vi "STED Control V13.vi"() -> ()   [LabVIEW 2014]
uses:
  Type Defs/Image Acquisition Parameters.ctl
  Laser Controls.ctl
  Detectors.ctl
  Type Defs/P541.ctl
  Type Defs/M227.ctl
  Type Defs/P612.ctl
  Type Defs/M686.ctl
  Type Defs/P841.ctl
  Type Defs/ASI.ctl
  Type Defs/N664_V2.ctl
  Type Defs/STED Graph Controls.ctl
  Type Defs/Display Controls.ctl
  Type Defs/Z comp.ctl
  FPGA-7842R-Reference.ctl
  Manual Controls V2.ctl
  Scan Parameters.ctl
  <vilib>/Utility/miscctls.llb/LVPositionTypeDef.ctl
  Controls/StageStates.ctl
  DM_Dual_V2/Controls/Standard Action.ctl
  Focus Lock/Controls/Counter Action.ctl
  Focus Lock/Controls/Standard Action for Focus Lock.ctl
  <vilib>/Utility/miscctls.llb/LVRectTypeDef.ctl
  <vilib>/event_ctls.llb/lveventtype.ctl
  <vilib>/Utility/file.llb/Read From Spreadsheet File (DBL).vi
  <vilib>/Utility/file.llb/Write To Spreadsheet File (DBL).vi
panel:
  in  "z Comp.":T1
  out "Graph Ref Out":refnum<vi>[](array[refnum])
  out "Frame Counter":i32
  in  "Follow Cursor":bool
  in  "Laser Controls 2":T2={"Laser On Time (Ticks)"=16, "Laser Delay (Ticks)"=3}
  out "Channel 6":sgl[][](graph)
  out "Channel 5":sgl[][](graph)
  out "Channel 4":sgl[][](graph)
  out "Channel 3":sgl[][](graph)
  out "Channel 2":sgl[][](graph)
  out "Channel 1":sgl[][](graph)
  in  "Display Controls":T3
  in  "Graph Tools":T4={"Zoom Out"=FALSE, "Zoom In"=FALSE, "Reset Zoom"=FALSE, "Pan Tool"=FALSE, "Show Cursor"=FALSE, "Load File"=FALSE, "Fit Tool"=FALSE, "Smooth Tool"=FALSE, "Merge Tool"=FALSE, "Auto Scale"=FALSE, "Apply Color"=FALSE, "Color Map"=enum."Fire"}
  in  "Shutters":T5
  in  "Upper Objective Z - N664":T6={"Up N664"=FALSE, "Down N664"=FALSE, "Step Size (um)"=0.001, "Position (mm)"=0.0, "Home"=FALSE, "Save"=FALSE} {"Step Size (um)" min=0.001}
  in  "Cavity Translation Z - ASI":T7={"Up ASI"=FALSE, "Down ASI"=FALSE, "Step Size (um)"=0.001, "Z (um)"=0.001, "F (um)"=0.001, "Velocity"=0.001} caption="ASI" {"Velocity" min=0.001; "F (um)" min=0.001; "Z (um)" min=-1500.0 max=1500.0; "Step Size (um)" min=0.001}
  in  "Phase Comp Mirror - P841":T8={"Position (µm)"=0.0, "Step Size (µm)"=0.05, "Up P841"=FALSE, "Down P841"=FALSE}
  in  "Sample Stage XY - M686":T9={"Home Button"=FALSE, "Up Button"=FALSE, "Left Button"=FALSE, "Down Button"=FALSE, "Right Button"=FALSE, "X"=0.0, "Y"=0.0, "Step Size (um)"=1.0} {"Y" format="%#_8g"; "X" format="%#_8g"}
  in  "Bottom Objective XY - P612":T10
  in  "Abort AllStage":bool
  in  "Stages":T11={"M227"=TRUE, "N664"=TRUE, "P612"=TRUE, "M686"=TRUE, "P841"=TRUE, "ASI"=FALSE}
  in  "Sample Z Coarse - M227":T12
  in  "Tab Control":T13(tab)
  in  "SLM":bool
  in  "DM":bool
  in  "Timing":bool
  in  "Focus Lock":bool
  in  "Stage Monitor":bool
  in  "Camera":bool
  in  "Sample Z - P541":T14={"Step Up"=FALSE, "Step Down"=FALSE, "Z Position"=0.0, "Step Size (um)"=1.0, "Home"=FALSE, "Save"=FALSE}
  in  "Detectors":T15={"PMT"=TRUE, "Far Red (685/40 nm)"=FALSE, "Orange (624/40 nm)"=FALSE, "Green (525/50 nm)"=FALSE, "Sum All"=FALSE}
  in  "Laser Controls":T16 {"STED Power (V)" scale=0.0..10.0}
  in  "Save File Path":path=path "C:/isoSTED_Data/Temp/Test_0000.dbl"
  in  "Capture":bool
  in  "Image Acquisition Parameters":T17={"Scan Type"=enum."Beam Scanning", "Scan Mode"=enum."XY", "Fast Axis Frequency (Hz)"=15780.0, "Image Format"=256, "Line Accumulations"=100, "Frames Per Capture"=1, "Frames Accumulations"=1, "Image Dimension (um)"=[15.0, 15.0], "Number of Z Steps"=1, "Z Steps Size (um)"=1.0, "Pixel Size (nm)"=[58.59375, 58.59375], "Customized Image Format"=[]} {"Z Steps Size (um)" min=0.0; "Number of Z Steps" min=1; "Frames Accumulations" min=1; "Frames Per Capture" min=1; "Line Accumulations" min=1; "Image Format" items=["64 x 64"=64, "128 x 128"=128, "256 x 256"=256, "512 x 512"=512, "1024 x 1024"=1024, "2048 x 2048"=2048, "Customized..."=0]}
  in  "Live":bool
  in  "Exit":bool
  # "Piston"
  # "Defocus"
  # "Length"
  # "Height"
  # "XY"
  # "Z"
  # "Length"
  # "Height"
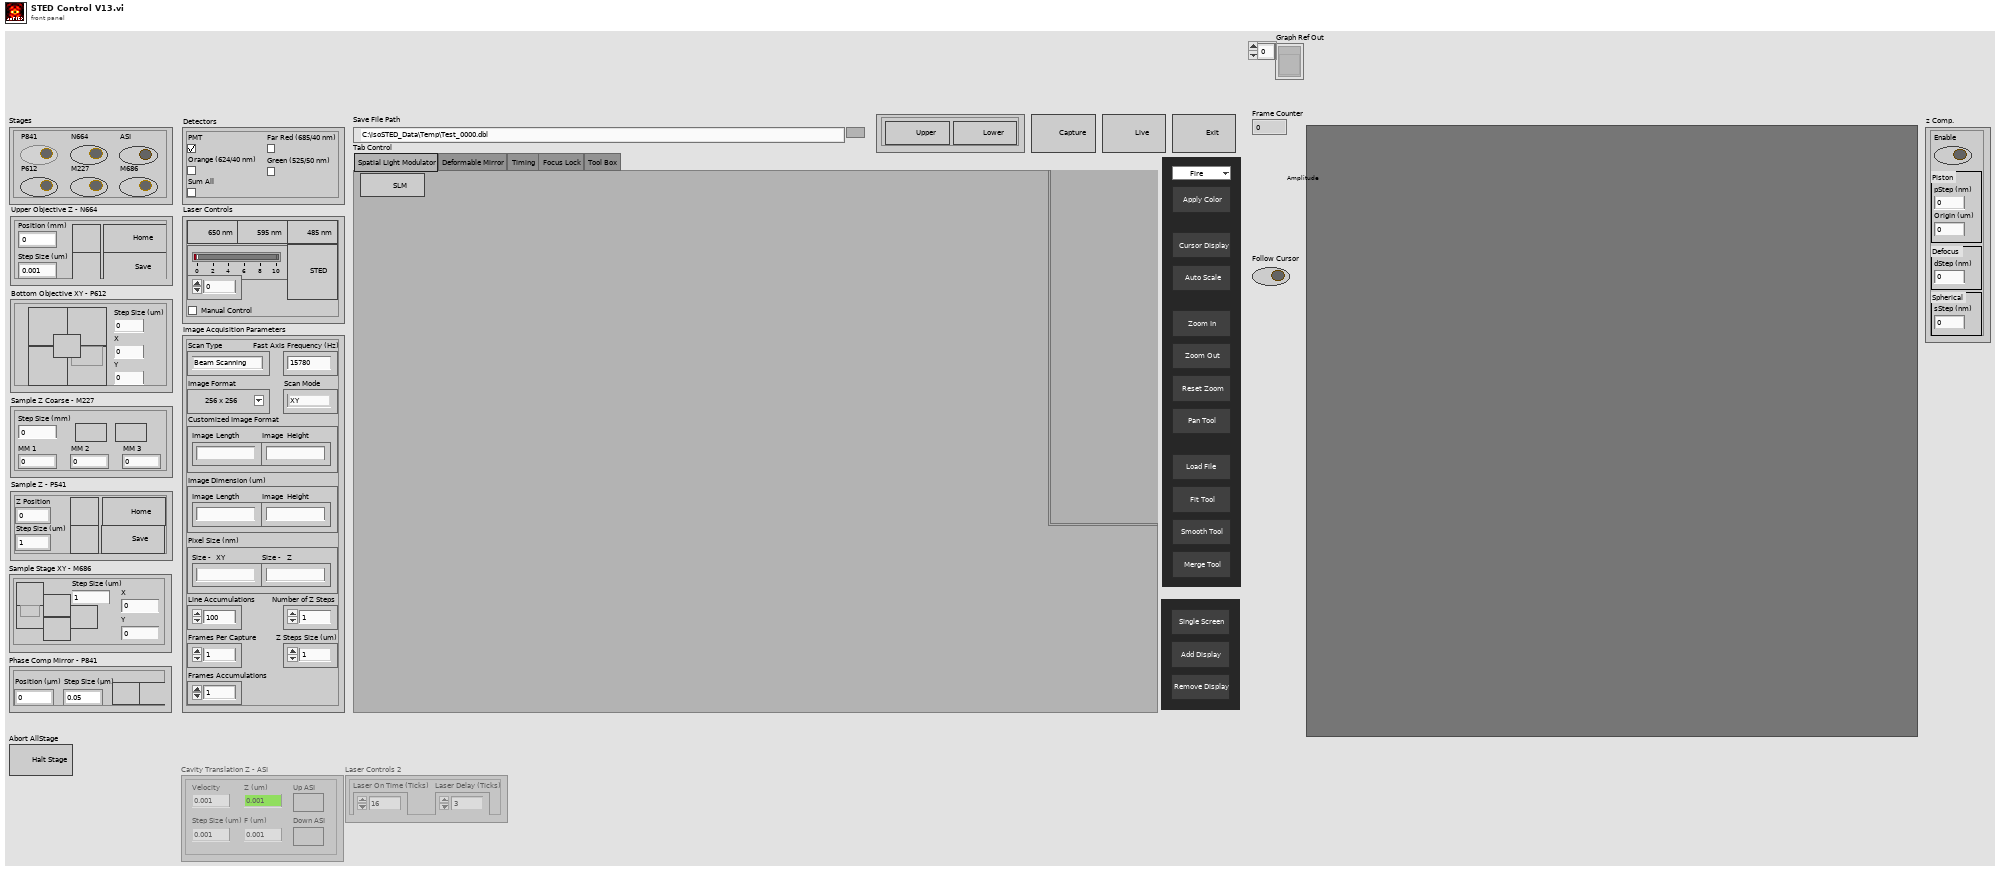
[diagram p1: front panel]
types:
  T1 = typedef "Z comp.ctl" = cluster{"Enable":bool, "pStep (nm)":dbl, "Origin (um)":dbl, "dStep (nm)":dbl, "sStep (nm)":dbl}
  T2 = cluster{"Laser On Time (Ticks)":i8, "Laser Delay (Ticks)":i8}
  T3 = typedef "Display Controls.ctl" = cluster{"Remove Display":bool, "Add Display":bool, "Single Screen":bool}
  T4 = typedef "STED Graph Controls.ctl" = cluster{"Zoom Out":bool, "Zoom In":bool, "Reset Zoom":bool, "Pan Tool":bool, "Show Cursor":bool, "Load File":bool, "Fit Tool":bool, "Smooth Tool":bool, "Merge Tool":bool, "Auto Scale":bool, "Apply Color":bool, "Color Map":enum16{"System", "Fire", "Gray", "Red", "Green", "Blue", "Cyan", "Magenta", "Yellow", "Red-White", "Green-White", "Blue-White", "Glow"}}
  T5 = cluster{"Upper Shutter":bool, "Lower Shutter":bool}
  T6 = typedef "N664_V2.ctl" = cluster{"Up N664":bool, "Down N664":bool, "Step Size (um)":dbl, "Position (mm)":dbl, "Home":bool, "Save":bool}
  T7 = typedef "ASI.ctl" = cluster{"Up ASI":bool, "Down ASI":bool, "Step Size (um)":dbl, "Z (um)":dbl, "F (um)":dbl, "Velocity":dbl}
  T8 = typedef "P841.ctl" = cluster{"Position (µm)":dbl, "Step Size (µm)":dbl, "Up P841":bool, "Down P841":bool}
  T9 = typedef "M686.ctl" = cluster{"Home Button":bool, "Up Button":bool, "Left Button":bool, "Down Button":bool, "Right Button":bool, "X":dbl, "Y":dbl, "Step Size (um)":dbl}
  T10 = typedef "P612.ctl" = cluster{"Home Button":bool, "Up Button":bool, "Left Button":bool, "Down Button":bool, "Right Button":bool, "Step Size (um)":dbl, "X":dbl, "Y":dbl}
  T11 = cluster{"M227":bool, "N664":bool, "P612":bool, "M686":bool, "P841":bool, "ASI":bool}
  T12 = typedef "M227.ctl" = cluster{"Up M227":bool, "Down M227":bool, "Step Size (mm)":dbl, "MM 1":dbl, "MM 2":dbl, "MM 3":dbl}
  T13 = enum32{"Spatial Light Modulator", "Deformable Mirror", "Timing", "Focus Lock", "Tool Box"}
  T14 = typedef "P541.ctl" = cluster{"Step Up":bool, "Step Down":bool, "Z Position":dbl, "Step Size (um)":dbl, "Home":bool, "Save":bool}
  T15 = typedef "Detectors.ctl" = cluster{"PMT":bool, "Far Red (685/40 nm)":bool, "Orange (624/40 nm)":bool, "Green (525/50 nm)":bool, "Sum All":bool}
  T16 = typedef "Laser Controls.ctl" = cluster{"STED Power (V)":dbl, "STED":bool, "650 nm":bool, "590 nm":bool, "485 nm":bool, "Manual Control":bool}
  T17 = typedef "Image Acquisition Parameters.ctl" = cluster{"Scan Type":enum16{"Sample Scanning", "Beam Scanning"}, "Scan Mode":enum16{"XY", "XZ", "YZ", "XYZ"}, "Fast Axis Frequency (Hz)":dbl, "Image Format":u16, "Line Accumulations":u16, "Frames Per Capture":u16, "Frames Accumulations":u16, "Image Dimension (um)":dbl[], "Number of Z Steps":u8, "Z Steps Size (um)":dbl, "Pixel Size (nm)":dbl[], "Customized Image Format":dbl[]}
  T18 = typedef "Scan Parameters.ctl" = cluster{"Fast_Ax_Amp_V":dbl, "Fast_Ax_Off_V":dbl, "Slow_Ax_Amp_V":dbl, "Slow_Ax_Off_V ":dbl, "Slow_Ax_Max_V_VperS":dbl, "Slow_Ax1_Del25ns":i32, "Slow_Ax2_Del25ns":i32, "Stage_X_Off_V":dbl, "Stage_Y_Off_V":dbl, "Stage_Z_Off_V":dbl, "Galvo1_Off_V":dbl, "Galvo2_Off_V":dbl, "Last_Scan_Mode":enum16{"XY", "XZ", "YZ", "XYZ"}, "Current_Scan_Mode":enum16{"XY", "XZ", "YZ", "XYZ"}, "Fly_Back_Lines":u16, "Linear_Ramp_End":u32, "Z_Step_I16":i16, "Z_Start_I16":i16, "Laser_States _U32":u32, "590_Voltage_I16":i16, "775_AOM_Volt_I16":i16, "Blanking OFF":bool, "Unused_Axis_I16":i16}
  T19 = typedef "Manual Controls V2.ctl" = cluster{"Galvo 1 Position (I16)":i16, "Galvo 2 Position (I16)":i16, "X Axis Voltage (I16)":i16, "Y Axis Voltage (I16)":i16, "Z Axis Voltage (I16)":i16, "Res Mirror Amp (I16)":i16, "Res Mirror Mute":bool, "Upper Shutter":bool, "Lower Shutter":bool}
  T20 = typedef "FPGA-7842R-Reference.ctl" = enum16{"Stage Control", "Laser Control", "Unused Axis I16", "Exit", "Set Res Mirror", "Set Galvo", "Current Frame for Capture", "Default", "Close FPGA", "Stop Waveforms", "Start Waveforms", "Shutter Control", "Initialize"}
  T21 = typedef "Counter Action.ctl" = enum16{"Zero", "Plus One", "Read"}
  T22 = typedef "StageStates.ctl" = enum16{"POSITION", "MVR", "MOVE", "HALT", "ONTARGET", "ERROR", "EXIT", "HOME", "ZEROPOS", "NANOPOS", "QUIT", "ANALOG"}
  T23 = enum8{"Enabled", "Disabled", "Disabled and Grayed Out"}
  T24 = typedef "Standard Action.ctl" = enum16{"Read", "Write"}
  T25 = typedef "Standard Action for Focus Lock.ctl" = enum16{"Read", "Write"}
  T26 = typedef "LVRectTypeDef.ctl" = cluster{"Left":i16, "Top":i16, "Right":i16, "Bottom":i16}
  T27 = enum32{"Invalid", "Standard", "Closed", "Hidden", "Minimized", "Maximized"}
  T28 = typedef "lveventtype.ctl" = enum32{"Null", "Timeout", "Annotation Menu Selection", "Annotation Menu Selection?", "App Instance Close", "App Instance Close?", "Autoscale Range Change", "Bookmark Info Change", "Cell Edit", "Cell Edit?", "Cursor Grab", "Cursor Grab?", "Cursor Menu Selection", "Cursor Menu Selection?", "Cursor Move", "Cursor Release", "Data Change", "Direction Change", "Display State Change", "Drag Ended", "Drag Enter", "Drag Leave", "Drag Over", "Drag Source Update", "Drag Starting", "Drag Starting?", "Drop", "Exec State Change", "Key Down", "Key Down?", "Key Repeat", "Key Repeat?", "Key Up", "Listbox Double Click", "Menu Activation?", "Menu Selection (App)", "Menu Selection? (App)", "Menu Selection (User)", "Mouse Down", "Mouse Down?", "Mouse Enter", "Mouse Leave", "Mouse Move", "Mouse Up", "Mouse Wheel", "NI Security User Change (App)", "Pane Size", "Panel Close", "Panel Close?", "Panel Resize", "Plot Attribute Change", "Scale Range Change", "Shortcut Menu Activation?", "Shortcut Menu Selection (App)", "Shortcut Menu Selection? (App)", "Shortcut Menu Selection (User)", "Tree Double Click", "Tree Drag", "Tree Drag?", "Tree Drop", "Tree Drop?", "Tree Item Close", "Tree Item Close?", "Tree Item Open", "Tree Item Open?", "User Event", "Value Change"}
  T29 = typedef "LVPositionTypeDef.ctl" = cluster{"Left":i32, "Top":i32}
  T30 = cluster{"Upper Shutter":bool, "Upper Shutter":bool}
  T31 = cluster{bool, bool, dbl, "Numeric":dbl, "Numeric":dbl, "Numeric":dbl}
  T32 = cluster{"Down_N664":bool, "Down_N664":bool, "Step Size (um)":dbl, "Numeric":dbl, bool, bool}
  T33 = cluster{bool, bool, bool, bool, bool, dbl, "Numeric":dbl, "Numeric":dbl}
  T34 = cluster{bool, bool, bool, bool, bool, "Numeric":dbl, "Numeric":dbl, dbl}
  T35 = cluster{"Enable":bool, "pStep (nm)":bool, "Origin (um)":bool, "dStep (nm)":bool, "sStep (nm)":bool}
  T36 = typedef "MirrorModes_DUAL.ctl" = cluster{"Mode":string, "Amplitude":dbl}[][]
  T37 = cluster{"Scan Type":bool, "Scan Mode":bool, "Fast Axis Frequency (Hz)":bool, "Image Format":bool, "Line Accumulations":bool, "Frames Per Capture":bool, "Frames Accumulations":bool, "Image Dimension (um)":bool[], "Number of Z Steps":bool, "Z Steps Size (um)":bool, "Pixel Size (nm)":bool[], "Customized Image Format":bool[]}
  T38 = typedef "Focus Lock.ctl" = cluster{"EXIT":bool, "Lock Current":bool, "Manual":bool, "Drift":bool, "Move":bool, "Control Option":bool}
  T39 = typedef "LVAllMonitorsDisplayTypeDef.ctl" = cluster{"Bounds":cluster{"Left":i16, "Top":i16, "Right":i16, "Bottom":i16}, "Depth":i16}[]
  T40 = cluster{"Bounds":cluster{"Left":i16, "Top":i16, "Right":i16, "Bottom":i16}, "Depth":i16}
  T41 = enum16{"System", "Fire", "Gray", "Red", "Green", "Blue", "Cyan", "Magenta", "Yellow", "Red-White", "Green-White", "Blue-White", "Glow"}
  T42 = typedef "LVPointDoubleTypeDef.ctl" = cluster{"Cursor X":dbl, "Cursor Y":dbl}
  T43 = typedef "LVRangeTypeDef.ctl" = cluster{"Minimum":dbl, "Maximum":dbl, "Increment":dbl, "Minor Increment":dbl, "Start":dbl}
  T44 = typedef "IMAQ Image.ctl" = refnum<image>
  T45 = typedef "Waveform Data.ctl" = cluster{"Waveform Scan Parameters":cluster{"Scanning Mode":u8, "Fast Axis WF Length (Elements)":i32, "Fast Axis Sample Period (Ticks)":u32, "Slow Axis 1 WF Length (Elements)":i32, "Slow Axis 1 Sample Period (Ticks)":u32, "Slow Axis 1 Delay (25 ns) Steps":i32, "Slow Axis 2 WFLength (Elements)":i32, "Slow Axis 2 Sample Period (Ticks)":u32, "Slow Axis 2 Delay (25 ns) Steps":i32}, "Fast Axis Waveform":dbl[], "Slow Axis 1 Waveform":dbl[], "Slow Axis 2 Waveform":dbl[]}
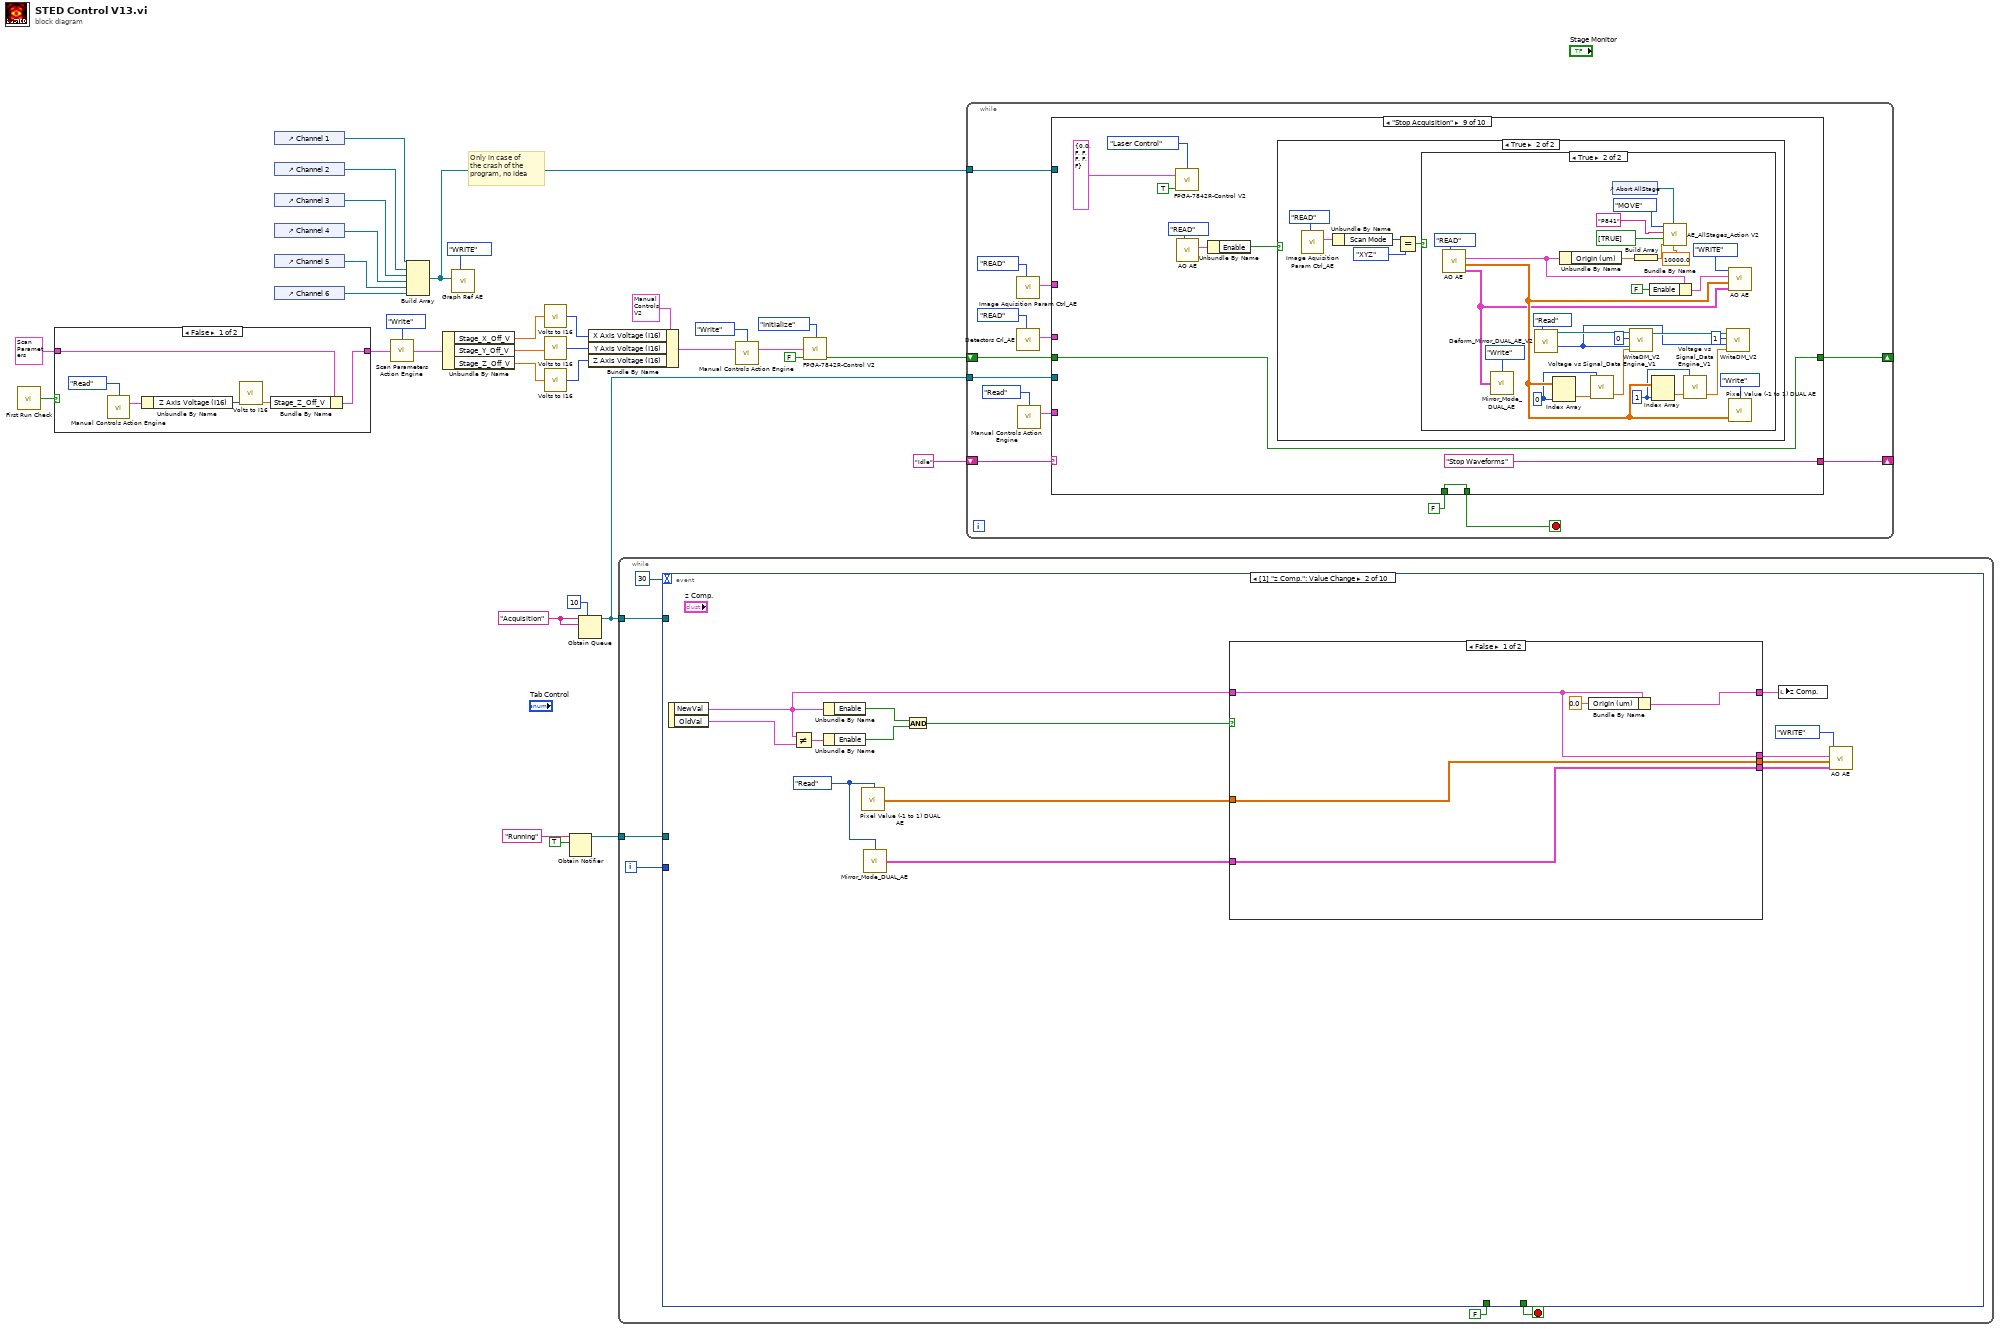
[diagram p0: block diagram]
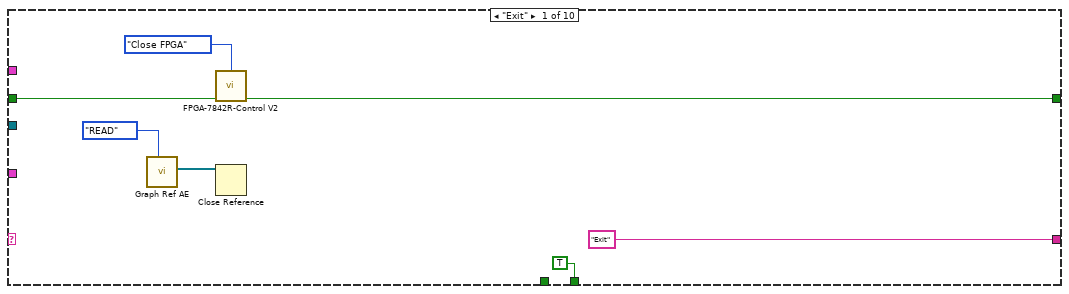
[diagram p3: hidden frame]
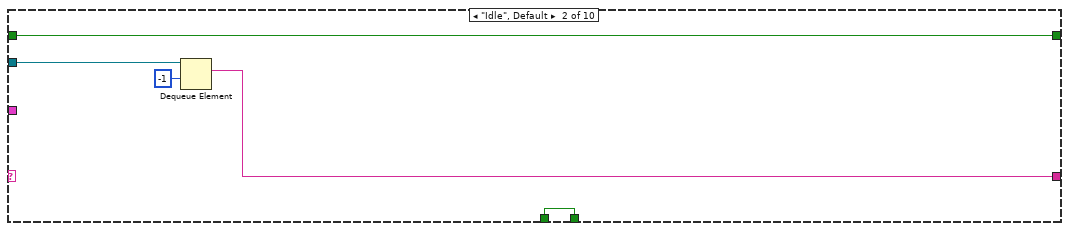
[diagram p4: hidden frame]
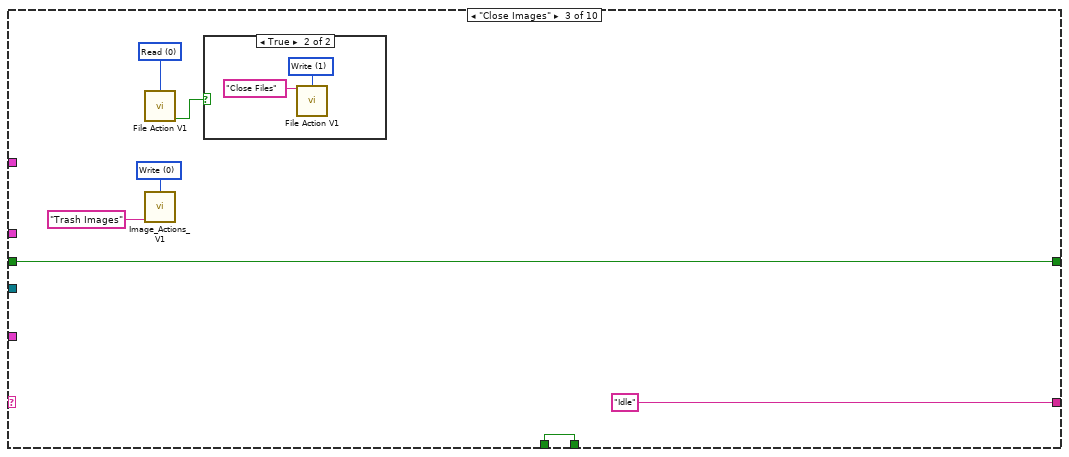
[diagram p5: hidden frame]
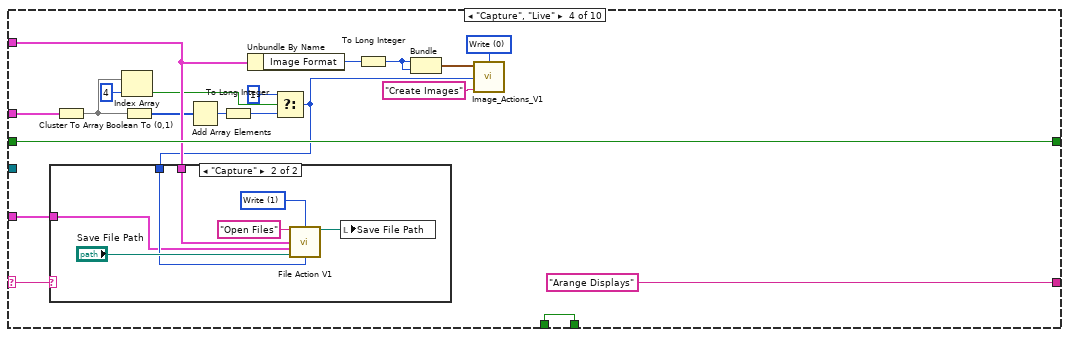
[diagram p7: hidden frame]
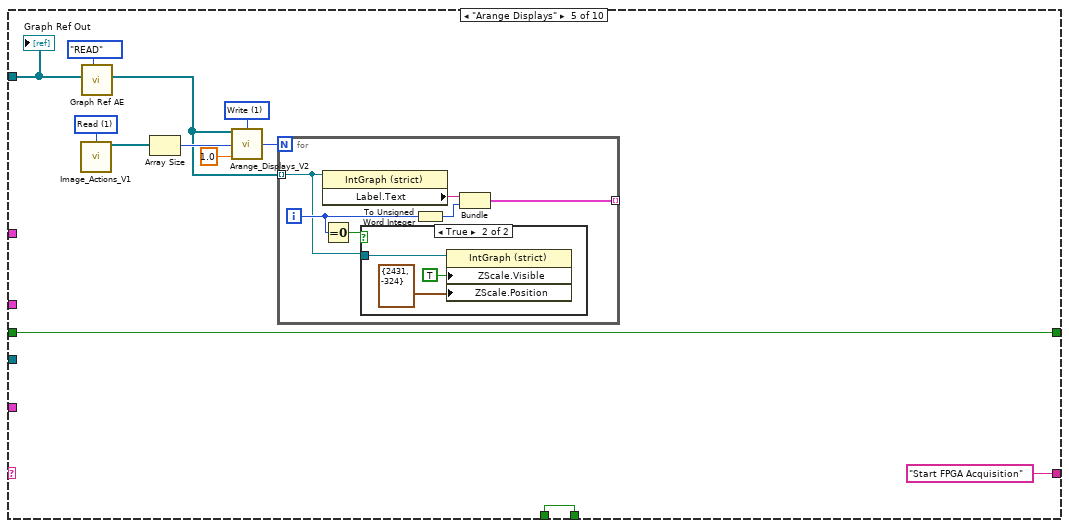
[diagram p9: hidden frame]
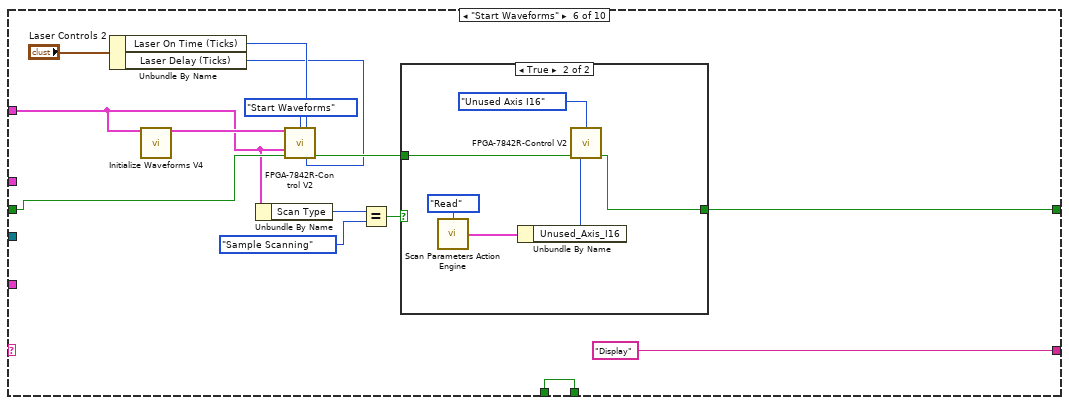
[diagram p11: hidden frame]
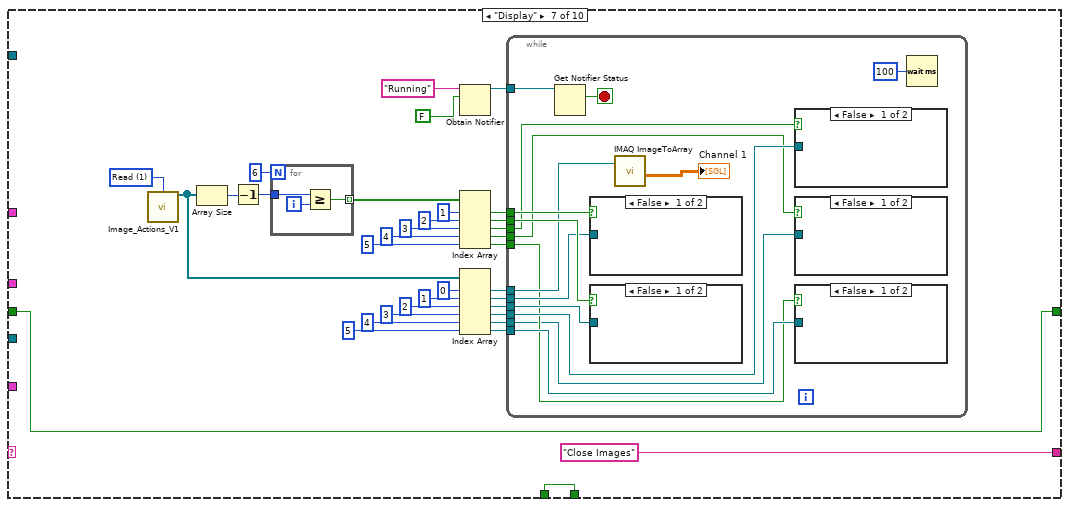
[diagram p13: hidden frame]
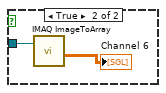
[diagram p14: hidden frame]
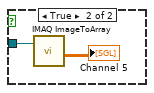
[diagram p15: hidden frame]
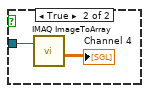
[diagram p16: hidden frame]
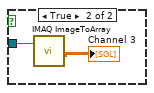
[diagram p17: hidden frame]
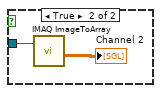
[diagram p18: hidden frame]
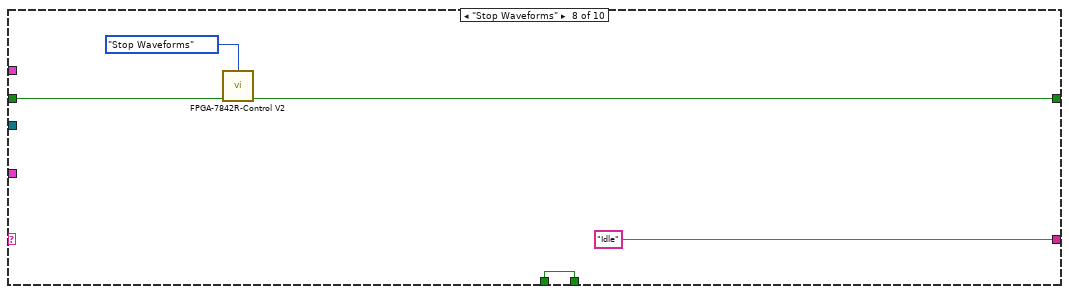
[diagram p19: hidden frame]
diagram:
  w16 = "Acquisition" ("name (unnamed)")
  # "Only in case of \nthe crash of the\nprogram, no idea"
  n1 = call "First Run Check.vi"() -> ("First Run?"=w10:bool)  [unwired: 15 in]
  n2 = case shown="False" w10 {
    tunnel: T18 {"Fast_Ax_Amp_V"=0.0, "Fast_Ax_Off_V"=0.0, "Slow_Ax_Amp_V"=0.0, "Slow_Ax_Off_V "=0.0, "Slow_Ax_Max_V_VperS"=0.0, "Slow_Ax1_Del25ns"=0, "Slow_Ax2_Del25ns"=0, "Stage_X_Off_V"=5.0, "Stage_Y_Off_V"=5.0, "Stage_Z_Off_V"=5.0, "Galvo1_Off_V"=0.0, "Galvo2_Off_V"=0.0, "Last_Scan_Mode"=enum."XY", "Current_Scan_Mode"=enum."XY", "Fly_Back_Lines"=0, "Linear_Ramp_End"=0, "Z_Step_I16"=0, "Z_Start_I16"=0, "Laser_States _U32"=0, "590_Voltage_I16"=0, "775_AOM_Volt_I16"=0, "Blanking OFF"=FALSE, "Unused_Axis_I16"=16384} ("Scan Parameters IN") -> [w39 w40]
    tunnel: [w34 w40] -> w8
    frame False {
      n3 = call "Manual Controls Action Engine.vi"("Action"=enum16{"Read", "Write"}."Read") -> ("Manual Controls Out"=w37:T19)  [unwired: 14 in]
      n4 = Unbundle By Name(w37) -> ("Z Axis Voltage (I16)"=w38:i16)
      n5 = call "Volts to I16.vi"("Volatge (I16)"=w38) -> ("Voltage (V)"=w35:dbl)  [unwired: 13 in, 1 out]
      n6 = Bundle By Name(cluster=w39, "Stage_Z_Off_V"=w35) -> (w34:T18)
    }
    frame True {
    }
  }
  n7 = control-ref of="Channel 1"() -> (w5:refnum<vi>)
  n8 = control-ref of="Channel 2"() -> (w6:refnum<vi>)
  n9 = control-ref of="Channel 3"() -> (w7:refnum<vi>)
  n10 = control-ref of="Channel 4"() -> (w2:refnum<vi>)
  n11 = control-ref of="Channel 5"() -> (w4:refnum<vi>)
  n12 = control-ref of="Channel 6"() -> (w3:refnum<vi>)
  n13 = call "Scan Parameters Action Engine.vi"("Action"=enum16{"Read", "Write"}."Write", "Scan Parameters IN"=w8) -> ("Scan Parameters OUT"=w26:T18)  [unwired: 13 in]
  n14 = Build Array(w5, w6, w7, w2, w4, w3) -> (w1:refnum<vi>[])
  n15 = Unbundle By Name(w26) -> ("Stage_X_Off_V"=w22:dbl, "Stage_Y_Off_V"=w21:dbl, "Stage_Z_Off_V"=w20:dbl)
  n16 = call "Graph Ref AE.vi"("Action"=enum16{"READ", "WRITE"}."WRITE", "Graph Ref In"=w1) -> ()  [unwired: 9 in, 1 out]
  n17 = call "Volts to I16.vi"("Voltage (V)"=w22) -> ("I16"=w23:i16)  [unwired: 13 in, 1 out]
  n18 = call "Volts to I16.vi"("Voltage (V)"=w21) -> ("I16"=w24:i16)  [unwired: 13 in, 1 out]
  n19 = call "Volts to I16.vi"("Voltage (V)"=w20) -> ("I16"=w25:i16)  [unwired: 13 in, 1 out]
  n20 = Obtain Notifier(name (unnamed)="Running", notification data type=TRUE) -> (notifier out=w12:refnum<notifier>)  [unwired: 2 in, 2 out]
  n21 = Obtain Queue(max queue size (-1, unlimited)=10, name (unnamed)=w16, element data type=w16) -> (queue out=w18:refnum<queue>)  [unwired: 2 in, 2 out]
  n22 = Bundle By Name(cluster=T19 {"Galvo 1 Position (I16)"=-280, "Galvo 2 Position (I16)"=0, "X Axis Voltage (I16)"=16384, "Y Axis Voltage (I16)"=16384, "Z Axis Voltage (I16)"=16384, "Res Mirror Amp (I16)"=0, "Res Mirror Mute"=FALSE, "Upper Shutter"=FALSE, "Lower Shutter"=FALSE} ("Manual Controls"), "X Axis Voltage (I16)"=w23, "Y Axis Voltage (I16)"=w24, "Z Axis Voltage (I16)"=w25) -> (w27:T19)
  n23 = while {
    tunnel: w18 -> [w44]
    tunnel: w12 -> [w41]
    i -> [w42]
    stop <- w46 stop-if-true
    n24 = event shown="[1] \"z Comp.\": Value Change" {
      selector: _ -> [_ _ _ _ _ _ _ _ _ _]
      dyn-events: _ -> [_ _ _ _ _ _ _ _ _ _]
      timeout: 30 -> [_ _ _ _ _ _ _ _ _ _]
      tunnel: [w54 _ w258 w302 w467 _ w814 w909 w1113 w1166] -> w46
      tunnel: FALSE -> [w54 _ w258 w302 w467 _ w814 w909 w1113 _]
      tunnel: w44 -> [w51 _ w257 _ _ _ _ _ _ w1165]
      tunnel: w42 -> [w49 _ _ _ _ _ _ _ _ _]
      tunnel: w41 -> [w47 _ w255 _ _ _ _ _ _ w1159]
      event Timeout {
        n25 = event-data() -> ()  [unwired: 1 in, 3 out]
        n26 = Equal To 0?(x=w49) -> (x = 0?=w48:bool)
        n27 = Get Notifier Status(notifier=w47) -> (current notification=w53:bool)  [unwired: 1 in, 4 out]
        n28 = case shown="False" w48 {
          frame False {
            w64 = enum16{"WRITE", "READ", "HOME", "SAVE HOME"}."READ" ("Enum")
            n29 = call "AO AE.vi"("Action"=enum16{"READ", "WRITE"}."READ") -> ("Z Comp. Output"=w57:T1)  [unwired: 8 in, 2 out]
            n30 = Unbundle By Name(w57) -> ("Enable"=w62:bool, "Origin (um)"=w58:dbl, "pStep (nm)"=w59:dbl, "dStep (nm)"=w56:dbl, "sStep (nm)"=w55:dbl)
            n31 = call "Image Aquisition Param Ctrl_AE.vi"("Action"=enum16{"READ", "WRITE"}."READ") -> ("Image Acquisition Parameters Out"=w98:T17)  [unwired: 10 in]
            n32 = call "Detectors Crl_AE.vi"("Action"=enum16{"READ", "WRITE"}."READ") -> ("Detectors Parameters Out"=w99:T15)  [unwired: 10 in]
            n33 = call "LASERs_ Crl_AE.vi"("Action"=enum16{"READ", "WRITE"}."READ") -> ("Detectors Parameters Out"=w100:T16)  [unwired: 10 in]
            n34 = local write "z Comp."(w57) -> ()
            n35 = local write "Image Acquisition Parameters"(w98) -> ()
            n36 = local write "Detectors"(w99) -> ()
            n37 = local write "Laser Controls"(w100) -> ()
            n38 = call "Frame Counter.vi"("Action"=Counter_Action."Read") -> ("Num"=w63:i32)
            "Frame Counter" <- w63
            n39 = case shown="True" w62 {
              tunnel: w63 -> [_ w104]
              tunnel: w59 -> [_ w105]
              tunnel: w58 -> [_ w103]
              tunnel: w57 -> [_ _]
              tunnel: w56 -> [_ w102]
              tunnel: w55 -> [_ w101]
              frame False {
              }
              frame True {
                n40 = local read "Capture"() -> (w112:bool)
                n41 = local read "Live"() -> (w113:bool)
                n42 = call "Image Aquisition Param Ctrl_AE.vi"("Action"=enum16{"READ", "WRITE"}."READ") -> ("Image Acquisition Parameters Out"=w114:T17)  [unwired: 10 in]
                n43 = Or(x=w112, y=w113) -> (x .or. y?=w109:bool)
                n44 = Unbundle By Name(w114) -> ("Scan Mode"=w111:enum16{"XY", "XZ", "YZ", "XYZ"}, "Number of Z Steps"=w106:u8)
                n45 = Equal?(x=enum16{"XY", "XZ", "YZ", "XYZ"}."XYZ", y=w111) -> (x = y?=w108:bool)
                n46 = And(x=w109, y=w108) -> (x .and. y?=w107:bool)
                n47 = case shown="True" w107 {
                  tunnel: w104 -> [_ w125]
                  tunnel: w106 -> [_ w124]
                  tunnel: w105 -> [_ w123]
                  tunnel: w103 -> [_ w122]
                  tunnel: w102 -> [_ w117]
                  tunnel: w101 -> [_ w116]
                  frame False {
                  }
                  frame True {
                    n48 = Quotient & Remainder(x=w125, y=w124) -> (x-y*floor(x/y)=w118:i32)  [unwired: 1 out]
                    n49 = control-ref of="Abort AllStage"() -> (w120:refnum<vi>)
                    n50 = call "Defocus and Spherical Comp V2.vi"("Spherical Step"=w116, "Defocus Step"=w117, "Step #"=w118) -> ()  [unwired: 1 in]
                    n51 = call "Piston Comp.vi"("Abort"=w120, "Step Size"=w123, "Step #"=w118, "Original Position"=w122, "Action"=enum16{"MOVE", "BACK TO ORIGINE"}."MOVE") -> ("position"=w119:dbl)  [unwired: 5 in]
                    n52 = property on="Position (µm)" class="DigNum (strict)"("Value"=w119) -> ()  [unwired: 2 in, 2 out]
                  }
                }
              }
            }
            n53 = call "Stage_position_ae.vi"("StageID"="M686", "Enum"=w64) -> ("Position Out"=w74:dbl[])  [unwired: 8 in, 1 out]
            n54 = call "Stage_position_ae.vi"("StageID"="M227", "Enum"=w64) -> ("Position Out"=w81:dbl[])  [unwired: 8 in, 1 out]
            n55 = call "Stage_position_ae.vi"("StageID"="N664", "Enum"=w64) -> ("Position Out"=w67:dbl[])  [unwired: 8 in, 1 out]
            n56 = call "Stage_position_ae.vi"("StageID"="P841", "Enum"=w64) -> ("Position Out"=w88:dbl[])  [unwired: 8 in, 1 out]
            n57 = call "Stage_position_ae.vi"("StageID"="P612", "Enum"=w64) -> ("Position Out"=w65:dbl[])  [unwired: 8 in, 1 out]
            n58 = Index Array(array=w67, index=0) -> (element=w84:dbl)
            n59 = Index Array(array=w88, index=0) -> (element=w61:dbl)
            n60 = Index Array(array=w65, index #1=0 ("index"), index #2=1 ("index"), index #3=2 ("index")) -> (element #1=w94:dbl, element #2=w91:dbl, element #3=w89:dbl)
            n61 = Index Array(array=w74, index #1=0 ("index"), index #2=1 ("index")) -> (element #1=w71:dbl, element #2=w70:dbl)
            n62 = Index Array(array=w81, index #1=0 ("index"), index #2=1 ("index"), index #3=2 ("index")) -> (element #1=w78:dbl, element #2=w77:dbl, element #3=w76:dbl)
            n63 = property on="Position (µm)" class="DigNum (strict)"("Value"=w61) -> ()  [unwired: 2 in, 2 out]
            n64 = property on="Position (mm)" class="DigNum (strict)"("Value"=w84) -> ()  [unwired: 2 in, 2 out]
            n65 = property on="X" class="DigNum (strict)"("Value"=w94) -> ()  [unwired: 2 in, 2 out]
            n66 = property on="Y" class="DigNum (strict)"("Value"=w91) -> ()  [unwired: 2 in, 2 out]
            n67 = property on="X" class="DigNum (strict)"("Value"=w71) -> ()  [unwired: 2 in, 2 out]
            n68 = property on="MM 1" class="DigNum (strict)"("Value"=w78) -> ()  [unwired: 2 in, 2 out]
            n69 = property on="MM 2" class="DigNum (strict)"("Value"=w77) -> ()  [unwired: 2 in, 2 out]
            n70 = property on="Z Position" class="DigNum (strict)"("Value"=w89) -> ()  [unwired: 2 in, 2 out]
            n71 = property on="Y" class="DigNum (strict)"("Value"=w70) -> ()  [unwired: 2 in, 2 out]
            n72 = property on="MM 3" class="DigNum (strict)"("Value"=w76) -> ()  [unwired: 2 in, 2 out]
          }
          frame True {
            w127 = FALSE ("SLM")
            w129 = enum16{"WRITE", "READ", "HOME", "SAVE HOME"}."SAVE HOME" ("Enum")
            w141 = FALSE ("Upper Shutter")
            n73 = local read "Image Acquisition Parameters"() -> (w148:T17)
            n74 = local read "Laser Controls"() -> (w146:T16)
            n75 = local read "Detectors"() -> (w145:T15)
            n76 = Bundle("Upper Shutter"=w141, "Upper Shutter"=w141) -> (w142:T30)  [unwired: 1 in]
            n77 = property on="Shutters" class="Clust (strict)"("Value"=w142) -> ()  [unwired: 2 in, 2 out]
            n78 = call "Image Aquisition Param Ctrl_AE.vi"("Action"=enum16{"READ", "WRITE"}."WRITE", "Image Acquisition Parameters In"=w148) -> ()  [unwired: 9 in, 1 out]
            n79 = call "Detectors Crl_AE.vi"("Action"=enum16{"READ", "WRITE"}."WRITE", "Detectors Parameters In"=w145) -> ()  [unwired: 9 in, 1 out]
            n80 = call "LASERs_ Crl_AE.vi"("Action"=enum16{"READ", "WRITE"}."WRITE", "Detectors Parameters In"=w146) -> ()  [unwired: 9 in, 1 out]
            n81 = property on="Stages" class="Clust (strict)"() -> ("Controls[]"=w143:refnum<vi>[])  [unwired: 2 in, 2 out]
            n82 = for {
              tunnel: w143 -> [w153] mode=indexing
              n83 = property class="Ctl"(reference=w153) -> ("Label.Text"=w151:string, "Value"=w155:variant)  [unwired: 1 in, 2 out]
              n84 = Variant To Data(type=TRUE, Variant=w155) -> (data=w152:bool)  [unwired: 1 in, 1 out]
              n85 = call "All_Stages_Aloha.vi"("Aloha"=w152, "Stage ID"=w151) -> ("Position Out"=w150:dbl[])  [unwired: 9 in]
              n86 = case shown="\"M686\"" w151 {
                tunnel: w150 -> [_ w162 w170 w177 w186 w197 w207]
                frame "0", Default {
                }
                frame "M227" {
                  w166 = FALSE
                  n87 = Index Array(array=w162, index #1=0 ("index"), index #2=1 ("index"), index #3=2 ("index")) -> (element #1=w158:dbl, element #2=w157:dbl, element #3=w156:dbl)
                  n88 = Bundle(w166, w166, 0.0, "Numeric"=w158, "Numeric"=w157, "Numeric"=w156) -> (w164:T31)  [unwired: 1 in]
                  n89 = To Variant(anything=w164) -> (Variant=w163:variant)
                  n90 = property on="Sample Z Coarse - M227" class="Clust"("Value"=w163) -> ()  [unwired: 2 in, 2 out]
                }
                frame "N664" {
                  w167 = FALSE
                  w173 = FALSE ("Down_N664")
                  n91 = Index Array(array=w170, index=0) -> (element=w171:dbl)
                  n92 = Bundle("Down_N664"=w173, "Down_N664"=w173, "Step Size (um)"=1.0, "Numeric"=w171, w167, w167) -> (w169:T32)  [unwired: 1 in]
                  n93 = To Variant(anything=w169) -> (Variant=w168:variant)
                  n94 = property on="Upper Objective Z - N664" class="Clust"("Value"=w168) -> ()  [unwired: 2 in, 2 out]
                }
                frame "P612" {
                  w185 = FALSE
                  n95 = Index Array(array=w177, index #1=0, index #2=1, index #3=2 ("index")) -> (element #1=w182:dbl, element #2=w180:dbl, element #3=w175:dbl)
                  n96 = Bundle(w185, w185, w185, w185, w185, 1.0, "Numeric"=w182, "Numeric"=w180) -> (w181:T33)  [unwired: 1 in]
                  n97 = To Variant(anything=w181) -> (Variant=w176:variant)
                  n98 = property on="Bottom Objective XY - P612" class="Clust"("Value"=w176) -> ()  [unwired: 2 in, 2 out]
                  n99 = property on="Z Position" class="DigNum (strict)"("Value"=w175) -> ()  [unwired: 2 in, 2 out]
                }
                frame "M686" {
                  w195 = FALSE
                  n100 = Index Array(array=w186, index #1=0, index #2=1) -> (element #1=w190:dbl, element #2=w189:dbl)
                  n101 = Bundle(w195, w195, w195, w195, w195, "Numeric"=w190, "Numeric"=w189, 1.0) -> (w193:T34)  [unwired: 1 in]
                  n102 = To Variant(anything=w193) -> (Variant=w191:variant)
                  n103 = property on="Sample Stage XY - M686" class="Clust"("Value"=w191) -> ()  [unwired: 2 in, 2 out]
                  n104 = call "M686_timer.vi"("Reset"=TRUE) -> ()  [unwired: 1 out]
                }
                frame "P841" {
                  n105 = Index Array(array=w197, index=0) -> (element=w196:dbl)
                  n106 = property on="Position (µm)" class="DigNum (strict)"("Value"=w196) -> ()  [unwired: 2 in, 2 out]
                }
                frame "ASI" {
                  w203 = FALSE
                  n107 = Add Array Elements(numeric array=w207) -> (sum=w209:dbl)
                  n108 = Index Array(array=w207, index #1=0 ("index"), index #2=1 ("index")) -> (element #1=w202:dbl, element #2=w201:dbl)
                  n109 = Divide(x=w209, y=2000.0) -> ()  [unwired: 1 out]
                  n110 = Bundle By Name(cluster=T7 {"Up ASI"=FALSE, "Down ASI"=FALSE, "Step Size (um)"=0.001, "Z (um)"=0.001, "F (um)"=0.001, "Velocity"=0.001} ("Cavity Translation Z - ASI"), "Up ASI"=w203, "Down ASI"=w203, "Step Size (um)"=1.0, "Z (um)"=w202, "F (um)"=w201, "Velocity"=0.1) -> (w199:T7)
                  n111 = To Variant(anything=w199) -> (Variant=w200:variant)
                  n112 = property on="Cavity Translation Z - ASI" class="Clust"("Value"=w200) -> ()  [unwired: 2 in, 2 out]
                }
              }
            }
            n113 = call-poly <vilib>:"Read From Spreadsheet File.vi"("format (%.3f)"="%.4f", "number of rows (all:-1)"=1, "file path (dialog if empty)"=path "C:/Users/ED STED/Documents/Test Control Software/Host VIs/Stages/Stage Positions/home position.csv") -> ("first row"=w138:dbl[])  [unwired: 4 in, 4 out]
            n114 = Index Array(array=w138, index #1=0 ("index"), index #2=1 ("index")) -> (element #1=w134:dbl, element #2=w135:dbl)
            n115 = Build Array(w134) -> (w133:dbl[])
            n116 = Build Array(w135) -> (w131:dbl[])
            n117 = call "Stage_position_ae.vi"("Position In"=w133, "StageID"="P541", "Enum"=w129) -> ()  [unwired: 7 in, 2 out]
            n118 = call "Stage_position_ae.vi"("Position In"=w131, "StageID"="N664", "Enum"=w129) -> ()  [unwired: 7 in, 2 out]
            n119 = local write "Focus Lock"(w127) -> ()
            n120 = local write "SLM"(w127) -> ()
            n121 = local write "Timing"(w127) -> ()
            n122 = local write "DM"(w127) -> ()
            n123 = local write "Camera"(w127) -> ()
            n124 = call "Frame Counter.vi"("Action"=Counter_Action."Zero") -> ()  [unwired: 1 out]
          }
        }
        n125 = local read "Capture"() -> (w52:bool)
        n126 = And(x=w53, y=w52) -> (x .and. y?=w50:bool)
        n127 = case shown="False" w50 {
          tunnel: w51 -> [_ w215]
          frame False {
          }
          frame True {
            w213 = T23."Enabled" ("Disabled")
            n128 = local write "Capture"(FALSE ("Capture")) -> ()
            n129 = call "Frame Counter.vi"("Action"=Counter_Action."Zero") -> ()  [unwired: 1 out]
            n130 = Enqueue Element(queue=w215, element="Stop Acquisition" ("f")) -> ()  [unwired: 2 in, 3 out]
            n131 = property on="Live" class="Bool (strict)"("DisabledEnum"=w213) -> ()  [unwired: 2 in, 2 out]
            n132 = property on="Exit" class="Bool"("DisabledEnum"=w213) -> ()  [unwired: 2 in, 2 out]
          }
        }
      }
      event Value Change {
        w224 = Standard_Action."Read" ("Action")
        n133 = event-data() -> ("NewVal"=w225:T1, "OldVal"=w230:T1)  [unwired: 1 in]
        n134 = Not Equal?(x=w225, y=w230) -> (x != y?=w229:T35)
        n135 = Unbundle By Name(w225) -> ("Enable"=w228:bool)
        n136 = Unbundle By Name(w229) -> ("Enable"=w227:bool)
        n137 = call "Pixel Value (-1 to 1) DUAL AE.vi"("Action"=w224) -> ("Pixel Value (-1 to 1) Out"=w217:dbl[][])  [unwired: 14 in]
        n138 = call "Mirror_Mode_DUAL_AE.vi"("Action"=w224) -> ("Mirror Modes Out"=w223:T36)  [unwired: 14 in]
        n139 = And(x=w228, y=w227) -> (x .and. y?=w226:bool)
        n140 = case shown="False" w226 {
          tunnel: w225 -> [w234 w243]
          tunnel: w217 -> [w231 w236]
          tunnel: w223 -> [w235 w237]
          tunnel: [w232 w238] -> w222
          tunnel: [w234 w238] -> w220
          tunnel: [w231 w236] -> w219
          tunnel: [w235 w237] -> w218
          frame False {
            n141 = Bundle By Name(cluster=w234, "Origin (um)"=0.0) -> (w232:T1)
          }
          frame True {
            n142 = call "AE_AllStages_Action V2.vi"("Stage ID"="P841" ("StageID"), "Action"=StageStates."MVR") -> ("Position Out"=w239:dbl[])  [unwired: 7 in, 2 out]
            n143 = Index Array(array=w239, index=0) -> (element=w242:dbl)
            n144 = Bundle By Name(cluster=w243, "Origin (um)"=w242) -> (w238:T1)
          }
        }
        n145 = local write "z Comp."(w222) -> ()
        n146 = call "AO AE.vi"("Mirror Modes In"=w218, "DM Value Input"=w219, "Z Comp. Input"=w220, "Action"=enum16{"READ", "WRITE"}."WRITE") -> ()  [unwired: 5 in, 3 out]
      }
      event "Live", "Capture": Value Change {
        w247 = FALSE ("element")
        n147 = event-data() -> ("CtlRef"=w256:refnum<vi>, "NewVal"=w254:bool)  [unwired: 1 in]
        n148 = call "Detectors Crl_AE.vi"() -> ("Detectors Parameters Out"=w253:T15)  [unwired: 11 in]
        n149 = Unbundle By Name(w253) -> ("PMT"=w252:bool, "Far Red (685/40 nm)"=w251:bool, "Orange (624/40 nm)"=w250:bool, "Green (525/50 nm)"=w249:bool, "Sum All"=w248:bool)
        n150 = Build Array(w252, w251, w250, w249, w248, w247, w247, w247) -> (w246:bool[])
        n151 = Boolean Array To Number(Boolean array=w246) -> (number=w245:u32)
        n152 = case shown="1, Default" w245 {
          tunnel: w257 -> [_ w267]
          tunnel: w256 -> [_ w266]
          tunnel: w255 -> [_ w261]
          tunnel: w254 -> [_ w260]
          frame 0 {
            w259 = FALSE ("Live")
            n153 = call "Display Message to User"() -> ()  [unwired: 10 in, 2 out]
            n154 = local write "Capture"(w259) -> ()
            n155 = local write "Live"(w259) -> ()
          }
          frame 1, Default {
            n156 = Not(x=w260) -> (.not. x?=w264:bool)
            n157 = property class="Bool (strict)"(reference=w266) -> ("Label.Text"=w262:string)  [unwired: 1 in, 2 out]
            n158 = Send Notification(notification=w264, notifier=w261) -> ()  [unwired: 1 in, 2 out]
            n159 = Select(t=w262, s=w260, f="Stop Acquisition") -> (s? t:f=w263:string)
            n160 = case shown="\"Capture\"" w262 {
              tunnel: w260 -> [_ w269 w283]
              frame "False", Default {
              }
              frame "Live" {
                n161 = case shown="True" w269 {
                  tunnel: [T23."Enabled" ("Disabled") T23."Disabled and Grayed Out" ("Disabled")] -> w268
                  frame False {
                    n162 = call "Frame Counter.vi"("Action"=Counter_Action."Zero") -> ()  [unwired: 1 out]
                  }
                  frame True {
                    n163 = call "AO AE.vi"("Action"=enum16{"READ", "WRITE"}."READ") -> ("DM Value Output"=w274:dbl[][], "Z Comp. Output"=w273:T1)  [unwired: 8 in, 1 out]
                    n164 = Unbundle By Name(w273) -> ("Enable"=w272:bool)
                    n165 = call "Frame Counter.vi"("Action"=Counter_Action."Zero") -> ()  [unwired: 1 out]
                    n166 = case shown="True" w272 {
                      tunnel: w274 -> [_ w279]
                      tunnel: w273 -> [_ w278]
                      frame False {
                      }
                      frame True {
                        n167 = call "Mirror_Mode_DUAL_AE.vi"("Action"=Standard_Action."Read") -> ("Mirror Modes Out"=w281:T36)  [unwired: 14 in]
                        n168 = call "AO AE.vi"("Mirror Modes In"=w281, "DM Value Input"=w279, "Z Comp. Input"=w278, "Action"=enum16{"READ", "WRITE"}."WRITE") -> ()  [unwired: 5 in, 3 out]
                      }
                    }
                  }
                }
                n169 = property on="Capture" class="Bool (strict)"("DisabledEnum"=w268) -> ()  [unwired: 2 in, 2 out]
                n170 = property on="Exit" class="Bool"("DisabledEnum"=w268) -> ()  [unwired: 2 in, 2 out]
              }
              frame "Capture" {
                n171 = case shown="False" w283 {
                  tunnel: [T23."Enabled" ("Disabled") T23."Disabled and Grayed Out" ("Disabled")] -> w284
                  frame False {
                    n172 = call "AO AE.vi"("Action"=enum16{"READ", "WRITE"}."READ") -> ("DM Value Output"=w287:dbl[][], "Z Comp. Output"=w286:T1)  [unwired: 8 in, 1 out]
                    n173 = call "Frame Counter.vi"("Action"=Counter_Action."Zero") -> ()  [unwired: 1 out]
                    n174 = Unbundle By Name(w286) -> ("Enable"=w285:bool)
                    n175 = case shown="True" w285 {
                      tunnel: w287 -> [_ w292]
                      tunnel: w286 -> [_ w291]
                      frame False {
                      }
                      frame True {
                        n176 = call "Mirror_Mode_DUAL_AE.vi"("Action"=Standard_Action."Read") -> ("Mirror Modes Out"=w294:T36)  [unwired: 14 in]
                        n177 = call "AO AE.vi"("Mirror Modes In"=w294, "DM Value Input"=w292, "Z Comp. Input"=w291, "Action"=enum16{"READ", "WRITE"}."WRITE") -> ()  [unwired: 5 in, 3 out]
                      }
                    }
                  }
                  frame True {
                    n178 = call "Frame Counter.vi"("Action"=Counter_Action."Zero") -> ()  [unwired: 1 out]
                  }
                }
                n179 = property on="Live" class="Bool (strict)"("DisabledEnum"=w284) -> ()  [unwired: 2 in, 2 out]
                n180 = property on="Exit" class="Bool"("DisabledEnum"=w284) -> ()  [unwired: 2 in, 2 out]
              }
            }
            n181 = Enqueue Element(queue=w267, element=w263) -> ()  [unwired: 2 in, 3 out]
          }
        }
      }
      event "Shutters": Value Change {
        n182 = event-data() -> ("CtlRef"=w301:refnum<vi>, "NewVal"=w300:variant, "OldVal"=w299:variant)  [unwired: 1 in]
        n183 = property class="Clust"(reference=w301) -> ("Label.Text"=w298:string)  [unwired: 1 in, 2 out]
        n184 = case shown="\"Image Acquisition Parameters\"" w298 {
          tunnel: w300 -> [_ w317 _ _ _]
          tunnel: w299 -> [_ w315 _ _ _]
          frame Default {
          }
          frame "Image Acquisition Parameters" {
            n185 = Variant To Data(type="Image Acquisition Parameters", Variant=w317) -> (data=w314:T17)  [unwired: 1 in, 1 out]
            n186 = Variant To Data(type=w314, Variant=w315) -> (data=w313:T17)  [unwired: 1 in, 1 out]
            n187 = Not Equal?(x=w314, y=w313) -> (x != y?=w338:T37)
            n188 = Unbundle By Name(w338) -> ("Image Dimension (um)"=w323:bool[], "Image Format"=w321:bool, "Pixel Size (nm)"=w322:bool[], "Scan Mode"=w304:bool)
            n189 = Or Array Elements(Boolean array=w323) -> (logical OR=w327:bool)
            n190 = Or Array Elements(Boolean array=w322) -> (logical OR=w326:bool)
            n191 = Build Array(w327, w321, w326) -> (w325:bool[])
            n192 = Boolean Array To Number(Boolean array=w325) -> (number=w324:u32)
            n193 = case shown="1, 2" w324 {
              tunnel: w323 -> [_ w388 _]
              tunnel: w314 -> [w376 w381 w396]
              tunnel: [w376 w379 w394] -> w320
              tunnel: w322 -> [_ _ w393]
              tunnel: [w375 w378 w392] -> w319
              tunnel: [w374 w377 w391] -> w306
              frame 0, Default {
                n194 = Unbundle By Name(w376) -> ("Image Dimension (um)"=w375:dbl[], "Scan Mode"=w374:enum16{"XY", "XZ", "YZ", "XYZ"})
              }
              frame 1, 2 {
                # "Image Dimension or Format Change"
                n195 = Unbundle By Name(w381) -> ("Image Dimension (um)"=w387:dbl[], "Image Format"=w385:u16, "Scan Mode"=w377:enum16{"XY", "XZ", "YZ", "XYZ"})
                n196 = for {
                  tunnel: w388 -> [w390] mode=indexing
                  tunnel: w387 -> [w389] mode=indexing
                  tunnel: [w389] -> w386
                  stop <- w390 stop-if-true
                }
                n197 = To Double Precision Float(number=w385) -> (double precision float=w384:dbl)
                n198 = Build Array(w386, w386) -> (w378:dbl[])
                n199 = Divide(x=w378, y=w384) -> (x/y=w383:dbl[])
                n200 = Multiply(x=w383, y=1000.0) -> (x*y=w380:dbl[])
                n201 = Bundle By Name(cluster=w381, "Image Dimension (um)"=w378, "Pixel Size (nm)"=w380) -> (w379:T17)
              }
              frame 4 {
                # "Pixel Size Change"
                n202 = Unbundle By Name(w396) -> ("Pixel Size (nm)"=w402:dbl[], "Image Format"=w400:u16, "Scan Mode"=w391:enum16{"XY", "XZ", "YZ", "XYZ"})
                n203 = for {
                  tunnel: w393 -> [w404] mode=indexing
                  tunnel: w402 -> [w403] mode=indexing
                  tunnel: [w403] -> w401
                  stop <- w404 stop-if-true
                }
                n204 = Build Array(w401, w401) -> (w395:dbl[])
                n205 = To Double Precision Float(number=w400) -> (double precision float=w399:dbl)
                n206 = Multiply(x=w395, y=w399) -> (x*y=w398:dbl[])
                n207 = Multiply(x=w398, y=0.001) -> (x*y=w392:dbl[])
                n208 = Bundle By Name(cluster=w396, "Pixel Size (nm)"=w395, "Image Dimension (um)"=w392) -> (w394:T17)
              }
            }
            n209 = And(x=w304, y="Follow Cursor") -> (x .and. y?=w303:bool)
            n210 = case shown="True" w303 {
              tunnel: w306 -> [_ w348]
              frame False {
              }
              frame True {
                n211 = Not Equal?(x=w348, y=enum16{"XY", "XZ", "YZ", "XYZ"}."XZ") -> (x != y?=w346:bool)
                n212 = case shown="True" w346 {
                  frame False {
                    n213 = call "Y Slice.vi"() -> ("Y position"=w356:dbl)  [unwired: 1 in]
                    n214 = Build Array(0.0 ("element"), w356) -> (w354:dbl[])
                    n215 = call "AllStage_Limits_Array.vi"("Step(um)/Position(units)"=w354, "Axis"=bool[] [TRUE, TRUE, TRUE], "Stage ID"="M686", "MOVE/MVR"=enum16{"MOVE", "MVR"}."MVR") -> ("Positions"=w350:dbl[], "Boolean Array"=w351:bool[], "Stage ID"=w352:string)  [unwired: 4 in, 1 out]
                    n216 = call "AE_AllStages_Action V2.vi"("Velocity"=0.0, "Positions"=w350, "Axis"=w351, "Stage ID"=w352, "Action"=StageStates."MVR") -> ()  [unwired: 4 in, 3 out]
                  }
                  frame True {
                    n217 = call "Z Slice.vi"() -> ("Y position"=w370:dbl)  [unwired: 1 in]
                    n218 = call "Manual Controls Action Engine.vi"("Action"=enum16{"Read", "Write"}."Read") -> ("Manual Controls Out"=w365:T19)  [unwired: 14 in]
                    n219 = Multiply(x=w370, y=327.68) -> (x*y=w372:dbl)
                    n220 = Round To Nearest(number=w372) -> (nearest integer value=w371:dbl)
                    n221 = Unbundle By Name(w365) -> ("Z Axis Voltage (I16)"=w368:i16)
                    n222 = To Word Integer(number=w371) -> (16bit integer=w367:i16)
                    n223 = Add(x=w368, y=w367) -> (x+y=w366:i16)
                    n224 = Bundle By Name(cluster=w365, "Z Axis Voltage (I16)"=w366) -> (w364:T19)
                    n225 = call "Manual Controls Action Engine.vi"("Action"=enum16{"Read", "Write"}."Write", "Manual Controls In"=w364) -> ("Manual Controls Out"=w362:T19)  [unwired: 13 in]
                    n226 = call "FPGA-7842R-Control V2.vi"("Action"=FPGA-7842R-Reference."Stage Control", "Manual Controls"=w362, "Initialize"=TRUE) -> ()  [unwired: 11 in, 2 out]
                  }
                }
              }
            }
            n227 = Index Array(array=w319, index=0) -> (element=w343:dbl)
            n228 = Not Equal?(x=enum16{"XY", "XZ", "YZ", "XYZ"}."YZ" ("y"), y=w306) -> (x != y?=w328:bool)
            n229 = call "Res Mirror um to Volts.vi"("Image Size (um)"=w343) -> ("Voltage (V)"=w307:dbl)
            n230 = Select(t=15780.0, s=w328, f=200.0) -> (s? t:f=w331:dbl)
            n231 = In Range and Coerce(upper limit=5.0, x=w307, lower limit=0.0) -> (coerced(x)=w309:dbl)  [unwired: 1 out]
            n232 = call "Scan Parameters Action Engine.vi"("Action"=enum16{"Read", "Write"}."Read") -> ("Scan Parameters OUT"=w310:T18)  [unwired: 14 in]
            n233 = Bundle By Name(cluster=w310, "Fast_Ax_Amp_V"=w309) -> (w308:T18)
            n234 = Bundle By Name(cluster=w320, "Fast Axis Frequency (Hz)"=w331) -> (w330:T17)
            n235 = call "Volts to I16.vi"("Voltage (V)"=w309) -> ("I16"=w342:i16)  [unwired: 13 in, 1 out]
            n236 = call "Scan Parameters Action Engine.vi"("Action"=enum16{"Read", "Write"}."Write", "Scan Parameters IN"=w308) -> ()  [unwired: 13 in, 1 out]
            n237 = call "Manual Controls Action Engine.vi"("Action"=enum16{"Read", "Write"}."Read") -> ("Manual Controls Out"=w336:T19)  [unwired: 14 in]
            n238 = Bundle By Name(cluster=w336, "Res Mirror Amp (I16)"=w342, "Res Mirror Mute"=w328) -> (w334:T19)
            n239 = call "Image Aquisition Param Ctrl_AE.vi"("Action"=enum16{"READ", "WRITE"}."WRITE", "Image Acquisition Parameters In"=w330) -> ()  [unwired: 9 in, 1 out]
            n240 = call "FPGA-7842R-Control V2.vi"("Action"=FPGA-7842R-Reference."Set Res Mirror", "Manual Controls"=w334, "Initialize"=TRUE) -> ()  [unwired: 11 in, 2 out]
            n241 = call "Manual Controls Action Engine.vi"("Action"=enum16{"Read", "Write"}."Write", "Manual Controls In"=w334) -> ()  [unwired: 13 in, 1 out]
          }
          frame "Detectors" {
            n242 = call "Detectors Crl_AE.vi"("Action"=enum16{"READ", "WRITE"}."WRITE", "Detectors Parameters In"="Detectors") -> ()  [unwired: 9 in, 1 out]
          }
          frame "Laser Controls" {
            w419 = FALSE ("element")
            n243 = Unbundle By Name("Laser Controls") -> ("STED"=w425:bool, "650 nm"=w422:bool, "590 nm"=w423:bool, "485 nm"=w424:bool, "STED Power (V)"=w416:dbl, "Manual Control"=w408:bool)
            n244 = local read "Live"() -> (w411:bool)
            n245 = call "LASERs_ Crl_AE.vi"("Action"=enum16{"READ", "WRITE"}."WRITE", "Detectors Parameters In"="Laser Controls") -> ()  [unwired: 9 in, 1 out]
            n246 = Or(x=w411, y=w408) -> (x .or. y?=w410:bool)
            n247 = In Range and Coerce(upper limit=10.0, x=w416, lower limit=0.0) -> (coerced(x)=w413:dbl)  [unwired: 1 out]
            n248 = Build Array(w425, w422, w423, w424, w419, w419, w419, w419) -> (w421:bool[])
            n249 = case shown="True" w410 {
              tunnel: "Laser Controls" -> [_ w439]
              frame False {
              }
              frame True {
                n250 = call "FPGA-7842R-Control V2.vi"("Action"=FPGA-7842R-Reference."Laser Control", "Laser Controls"=w439, "Initialize"=TRUE) -> ()  [unwired: 11 in, 2 out]
              }
            }
            n251 = Boolean Array To Number(Boolean array=w421) -> (number=w420:u32)
            n252 = To Unsigned Byte Integer(number=w420) -> (unsigned 8bit integer=w418:u8)
            n253 = call "U8_To_U32.vi"("U8 IN"=w418) -> ("U32 OUT"=w417:u32)  [unwired: 13 in, 1 out]
            n254 = call "Volts to I16.vi"("Voltage (V)"=w413) -> ("I16"=w412:i16)  [unwired: 13 in, 1 out]
            n255 = case shown="False" w408 {
              tunnel: "Laser Controls" -> [w437 _]
              frame False {
                n256 = Unbundle By Name(w437) -> ("650 nm"=w434:bool, "590 nm"=w433:bool, "485 nm"=w432:bool)
                n257 = call "Detectors Crl_AE.vi"("Action"=enum16{"READ", "WRITE"}."READ") -> ("Detectors Parameters Out"=w435:T15)  [unwired: 10 in]
                n258 = Bundle By Name(cluster=w435, "Far Red (685/40 nm)"=w434, "Orange (624/40 nm)"=w433, "Green (525/50 nm)"=w432) -> (w431:T15)
                n259 = call "Detectors Crl_AE.vi"("Action"=enum16{"READ", "WRITE"}."WRITE", "Detectors Parameters In"=w431) -> ()  [unwired: 9 in, 1 out]
              }
              frame True {
              }
            }
            n260 = call "Scan Parameters Action Engine.vi"("Action"=enum16{"Read", "Write"}."Read") -> ("Scan Parameters OUT"=w428:T18)  [unwired: 14 in]
            n261 = Bundle By Name(cluster=w428, "Laser_States _U32"=w417, "775_AOM_Volt_I16"=w412) -> (w426:T18)
            n262 = call "Scan Parameters Action Engine.vi"("Action"=enum16{"Read", "Write"}."Write", "Scan Parameters IN"=w426) -> ()  [unwired: 13 in, 1 out]
          }
          frame "Shutters" {
            n263 = Unbundle By Name("Shutters") -> ("Upper Shutter"=w451:bool, "Lower Shutter"=w450:bool)
            n264 = Not(x=w451) -> (.not. x?=w442:bool)
            n265 = Not(x=w450) -> (.not. x?=w441:bool)
            n266 = call "Manual Controls Action Engine.vi"("Action"=enum16{"Read", "Write"}."Read") -> ("Manual Controls Out"=w446:T19)  [unwired: 14 in]
            n267 = Bundle By Name(cluster=w446, "Upper Shutter"=w442, "Lower Shutter"=w441) -> (w443:T19)
            n268 = call "Manual Controls Action Engine.vi"("Action"=enum16{"Read", "Write"}."Write", "Manual Controls In"=w443) -> ()  [unwired: 13 in, 1 out]
            n269 = call "FPGA-7842R-Control V2.vi"("Action"=FPGA-7842R-Reference."Shutter Control", "Manual Controls"=w443, "Initialize"=TRUE) -> ()  [unwired: 11 in, 2 out]
          }
        }
      }
      event Value Change {
        # "For P541 - Sample Z - Converting from Step in µm to I16 is as follows. We have (Step µw)*(10 V / 100 µm)*(32768 I16 / 10 V) = (Step µm)*(32768 I16 / 100 µm) = (Step µm)*(327.68 I16/µm)"
        n270 = event-data() -> ("CtlRef"=w465:refnum<vi>, "OldVal"=w463:variant, "NewVal"=w464:variant)  [unwired: 1 in]
        n271 = local write "Abort AllStage"(FALSE ("Abort AllStage")) -> ()
        n272 = property class="Clust"(reference=w465) -> ("Label.Text"=w462:string)  [unwired: 1 in, 2 out]
        n273 = case shown="\"Phase Comp Mirror - P841\"" w462 {
          tunnel: w464 -> [_ w488 w529 w556 w619 w660 w689 w728]
          tunnel: w463 -> [_ w487 w528 w555 w620 w661 w690 w729]
          tunnel: ["" "N664" "ASI" "P612" "P612" "P841" "M227" "M686"] -> w461
          tunnel: [dbl[] [0.0] w479 w521 w544 dbl[] [0.0] w649 w682 w718] -> w460
          tunnel: [bool[] [FALSE] w477 w515 w545 bool[] [FALSE] bool[] [TRUE] w683 w717] -> w459
          tunnel: [enum16{"MOVE", "MVR"}."MVR" ("MOVE/MVR") w476 w518 w547 enum16{"MOVE", "MVR"}."MVR" ("MOVE/MVR") w652 w675 w720] -> w458
          tunnel: [0.0 ("Step Size (um)") 0.5 ("Step Size (um)") w520 0.0 ("Velocity") 0.0 ("Velocity") 10000.0 ("Velocity") 0.0 ("Velocity") 0.0 ("Velocity")] -> w454
          tunnel: [StageStates."MVR" ("Action") w474 w519 w548 StageStates."POSITION" ("Action") w653 w679 w721] -> w452
          frame Default {
          }
          frame "Upper Objective Z - N664" {
            n274 = call "N664_Ctrl_Index.vi"("OldVal"=w487, "NewVal"=w488) -> ("Control Ref OUT"=w486:refnum<vi>, "N664 Out"=w484:T6)  [unwired: 12 in]
            n275 = property class="Ctl"(reference=w486) -> ("Label.Text"=w485:string)  [unwired: 1 in, 2 out]
            n276 = Unbundle By Name(w484) -> ("Step Size (um)"=w483:dbl, "Position (mm)"=w482:dbl)
            n277 = case shown="\"Home\"" w485 {
              tunnel: w483 -> [_ w493 w496 _ _ _]
              tunnel: [0.0 ("Step Size (um)") w492 w496 w501 w503 w508] -> w480
              tunnel: w482 -> [_ _ _ w501 w503 _]
              tunnel: [enum16{"MOVE", "MVR"}."MVR" ("MOVE/MVR") enum16{"MOVE", "MVR"}."MVR" ("MOVE/MVR") enum16{"MOVE", "MVR"}."MVR" ("MOVE/MVR") enum16{"MOVE", "MVR"}."MOVE" ("MOVE/MVR") enum16{"MOVE", "MVR"}."MOVE" ("MOVE/MVR") enum16{"MOVE", "MVR"}."MOVE" ("MOVE/MVR")] -> w476
              tunnel: [StageStates."MVR" ("Action") StageStates."MVR" ("Action") StageStates."MVR" ("Action") StageStates."MOVE" ("Action") StageStates."MOVE" ("Action") StageStates."MOVE" ("Action")] -> w474
              frame Default {
              }
              frame "Up N664" {
                n278 = Negate(x=w493) -> (-x=w492:dbl)
              }
              frame "Down N664" {
              }
              frame "Position (mm)" {
              }
              frame "Save" {
                n279 = Build Array(w503) -> (w502:dbl[])
                n280 = call "Stage_position_ae.vi"("Position In"=w502, "StageID"="N664", "Enum"=enum16{"WRITE", "READ", "HOME", "SAVE HOME"}."SAVE HOME") -> ()  [unwired: 7 in, 2 out]
              }
              frame "Home" {
                n281 = call "Stage_position_ae.vi"("StageID"="N664", "Enum"=enum16{"WRITE", "READ", "HOME", "SAVE HOME"}."HOME") -> ("Position Out"=w510:dbl[])  [unwired: 8 in, 1 out]
                n282 = Index Array(array=w510, index=0) -> (element=w508:dbl)
              }
            }
            n283 = Build Array(w480) -> (w479:dbl[])
            n284 = Build Array(TRUE) -> (w477:bool[])
          }
          frame "Cavity Translation Z - ASI" {
            n285 = call "ASI_Ctrl_Index.vi"("NewVal"=w529, "OldVal"=w528) -> ("ASI out"=w525:T7, "Control Ref OUT"=w527:refnum<vi>)  [unwired: 8 in]
            n286 = property class="Ctl"(reference=w527) -> ("Label.Text"=w526:string)  [unwired: 1 in, 2 out]
            n287 = Unbundle By Name(w525) -> ("Step Size (um)"=w524:dbl, "Z (um)"=w523:dbl, "Velocity"=w520:dbl)
            n288 = case shown="\"Z (um)\"" w526 {
              tunnel: w524 -> [_ w535 w538 _]
              tunnel: w523 -> [_ _ _ w542]
              tunnel: [0.0 ("Z (um)") w535 w539 w542] -> w522
              tunnel: [StageStates."MVR" ("Action") StageStates."MVR" ("Action") StageStates."MVR" ("Action") StageStates."MOVE" ("Action")] -> w519
              tunnel: [enum16{"MOVE", "MVR"}."MVR" ("MOVE/MVR") enum16{"MOVE", "MVR"}."MVR" ("MOVE/MVR") enum16{"MOVE", "MVR"}."MVR" ("MOVE/MVR") enum16{"MOVE", "MVR"}."MOVE" ("MOVE/MVR")] -> w518
              frame Default {
              }
              frame "Up ASI" {
              }
              frame "Down ASI" {
                n289 = Negate(x=w538) -> (-x=w539:dbl)
              }
              frame "Z (um)" {
              }
            }
            n290 = Build Array(w522) -> (w521:dbl[])
            n291 = Build Array(TRUE) -> (w515:bool[])
          }
          frame "Bottom Objective XY - P612" {
            n292 = call "P612_Ctrl_Index.vi"("OldVal"=w555, "NewVal"=w556) -> ("Control out"=w554:refnum<vi>, "P612 out"=w552:T10)  [unwired: 12 in]
            n293 = property class="Ctl"(reference=w554) -> ("Label.Text"=w553:string)  [unwired: 1 in, 2 out]
            n294 = Unbundle By Name(w552) -> ("Step Size (um)"=w551:dbl, "X"=w550:dbl, "Y"=w549:dbl)
            n295 = case shown="\"Up Button\"" w553 {
              tunnel: w551 -> [_ _ w567 w574 w578 w585 _]
              tunnel: w550 -> [_ _ _ _ _ _ w592]
              tunnel: w549 -> [_ _ _ _ _ _ w591]
              tunnel: [StageStates."MVR" ("Action") StageStates."HOME" ("Action") StageStates."MVR" ("Action") StageStates."MVR" ("Action") StageStates."MVR" ("Action") StageStates."MVR" ("Action") StageStates."MOVE" ("Action")] -> w548
              tunnel: [enum16{"MOVE", "MVR"}."MVR" ("MOVE/MVR") enum16{"MOVE", "MVR"}."MVR" ("MOVE/MVR") enum16{"MOVE", "MVR"}."MVR" ("MOVE/MVR") enum16{"MOVE", "MVR"}."MVR" ("MOVE/MVR") enum16{"MOVE", "MVR"}."MVR" ("MOVE/MVR") enum16{"MOVE", "MVR"}."MVR" ("MOVE/MVR") enum16{"MOVE", "MVR"}."MOVE" ("MOVE/MVR")] -> w547
              tunnel: [bool[] [FALSE] bool[] [TRUE, TRUE] bool[] [TRUE, FALSE] bool[] [TRUE, FALSE] bool[] [FALSE, TRUE] bool[] [FALSE, TRUE] bool[] [TRUE, TRUE]] -> w545
              tunnel: [dbl[] [0.0] dbl[] [0.0, 0.0] w566 w573 w580 w587 w593] -> w544
              frame Default {
              }
              frame "Home Button" {
              }
              frame "Up Button" {
                n296 = Build Array(w567, 0.0 ("element")) -> (w566:dbl[])
              }
              frame "Down Button" {
                n297 = Negate(x=w574) -> (-x=w571:dbl)
                n298 = Build Array(w571, 0.0 ("element")) -> (w573:dbl[])
              }
              frame "Left Button" {
                n299 = Build Array(0.0 ("element"), w578) -> (w580:dbl[])
              }
              frame "Right Button" {
                n300 = Negate(x=w585) -> (-x=w584:dbl)
                n301 = Build Array(0.0 ("element"), w584) -> (w587:dbl[])
              }
              frame "X", "Y" {
                n302 = Build Array(w592, w591) -> (w593:dbl[])
              }
            }
          }
          frame "Sample Z - P541" {
            w598 = 327.68 ("y")
            n303 = call "P541_Ctrl_Index.vi"("OldVal"=w620, "NewVal"=w619) -> ("Control out"=w618:refnum<vi>, "P541 Out"=w617:T14)  [unwired: 12 in]
            n304 = Unbundle By Name(w617) -> ("Z Position"=w597:dbl, "Step Size (um)"=w616:dbl)
            n305 = property class="Ctl"(reference=w618) -> ("Label.Text"=w615:string)  [unwired: 1 in, 2 out]
            n306 = call "Manual Controls Action Engine.vi"("Action"=enum16{"Read", "Write"}."Read") -> ("Manual Controls Out"=w606:T19)  [unwired: 14 in]
            n307 = Unbundle By Name(w606) -> ("Z Axis Voltage (I16)"=w609:i16)
            n308 = Multiply(x=w597, y=w598) -> (x*y=w612:dbl)
            n309 = Multiply(x=w616, y=w598) -> (x*y=w614:dbl)
            n310 = Round To Nearest(number=w612) -> (nearest integer value=w601:dbl)
            n311 = Round To Nearest(number=w614) -> (nearest integer value=w600:dbl)
            n312 = To Word Integer(number=w601) -> (16bit integer=w611:i16)
            n313 = To Word Integer(number=w600) -> (16bit integer=w613:i16)
            n314 = case shown="\"Home\"" w615 {
              tunnel: w613 -> [_ w627 w631 _ _ _]
              tunnel: w611 -> [_ _ _ w633 _ _]
              tunnel: w609 -> [w626 w629 w632 _ w638 _]
              tunnel: [w626 w628 w630 w633 w638 w644] -> w605
              tunnel: w598 -> [_ _ _ _ _ w643]
              tunnel: w597 -> [_ _ _ _ w637 _]
              frame Default {
              }
              frame "Step Down" {
                n315 = Subtract(x=w629, y=w627) -> (x-y=w628:i16)
              }
              frame "Step Up" {
                n316 = Add(x=w632, y=w631) -> (x+y=w630:i16)
              }
              frame "Z Position" {
              }
              frame "Save" {
                n317 = Build Array(w637) -> (w636:dbl[])
                n318 = call "Stage_position_ae.vi"("Position In"=w636, "StageID"="P541", "Enum"=enum16{"WRITE", "READ", "HOME", "SAVE HOME"}."SAVE HOME") -> ()  [unwired: 7 in, 2 out]
              }
              frame "Home" {
                n319 = call "Stage_position_ae.vi"("StageID"="P541", "Enum"=enum16{"WRITE", "READ", "HOME", "SAVE HOME"}."HOME") -> ("Position Out"=w641:dbl[])  [unwired: 8 in, 1 out]
                n320 = Index Array(array=w641, index=0) -> (element=w639:dbl)
                n321 = Multiply(x=w639, y=w643) -> (x*y=w645:dbl)
                n322 = Round To Nearest(number=w645) -> (nearest integer value=w646:dbl)
                n323 = To Word Integer(number=w646) -> (16bit integer=w644:i16)
              }
            }
            n324 = Bundle By Name(cluster=w606, "Z Axis Voltage (I16)"=w605) -> (w608:T19)
            n325 = call "Manual Controls Action Engine.vi"("Action"=enum16{"Read", "Write"}."Write", "Manual Controls In"=w608) -> ("Manual Controls Out"=w602:T19)  [unwired: 13 in]
            n326 = call "FPGA-7842R-Control V2.vi"("Action"=FPGA-7842R-Reference."Stage Control", "Manual Controls"=w602, "Initialize"=TRUE) -> ()  [unwired: 11 in, 2 out]
          }
          frame "Phase Comp Mirror - P841" {
            n327 = call "P841_Ctrl_Index.vi"("OldVal"=w661, "NewVal"=w660) -> ("Control out"=w658:refnum<vi>, "P841 Out"=w656:T8)  [unwired: 12 in]
            n328 = property class="Ctl"(reference=w658) -> ("Label.Text"=w657:string)  [unwired: 1 in, 2 out]
            n329 = Unbundle By Name(w656) -> ("Position (µm)"=w655:dbl, "Step Size (µm)"=w654:dbl)
            n330 = case shown="Default" w657 {
              tunnel: w655 -> [_ _ _ w674]
              tunnel: w654 -> [_ w667 w671 _]
              tunnel: [0.0 ("Position (µm)") w667 w670 w674] -> w650
              tunnel: [StageStates."MVR" ("Action") StageStates."MVR" ("Action") StageStates."MVR" ("Action") StageStates."MOVE" ("Action")] -> w653
              tunnel: [enum16{"MOVE", "MVR"}."MVR" ("MOVE/MVR") enum16{"MOVE", "MVR"}."MVR" ("MOVE/MVR") enum16{"MOVE", "MVR"}."MVR" ("MOVE/MVR") enum16{"MOVE", "MVR"}."MOVE" ("MOVE/MVR")] -> w652
              frame Default {
              }
              frame "Up P841" {
              }
              frame "Down P841" {
                n331 = Negate(x=w671) -> (-x=w670:dbl)
              }
              frame "Position (µm)" {
              }
            }
            n332 = Build Array(w650) -> (w649:dbl[])
          }
          frame "Sample Z Coarse - M227" {
            n333 = call "M227_Ctrl_Index.vi"("OldVal"=w690, "NewVal"=w689) -> ("Control Ref OUT"=w688:refnum<vi>, "M227 Out"=w686:T12)  [unwired: 12 in]
            n334 = property class="Ctl"(reference=w688) -> ("Label.Text"=w687:string)  [unwired: 1 in, 2 out]
            n335 = Unbundle By Name(w686) -> ("Step Size (mm)"=w685:dbl, "MM 1"=w678:dbl, "MM 2"=w677:dbl, "MM 3"=w676:dbl)
            n336 = case shown="\"MM 1\"" w687 {
              tunnel: w685 -> [_ _ _ _ w709 w714]
              tunnel: [bool[] [FALSE, FALSE, FALSE] bool[] [TRUE, TRUE, TRUE] bool[] [TRUE, TRUE, TRUE] bool[] [TRUE, TRUE, TRUE] bool[] [TRUE, TRUE, TRUE] bool[] [TRUE, TRUE, TRUE]] -> w683
              tunnel: [0.0 ("Step Size (mm)") w696 w700 w704 w709 w713] -> w680
              tunnel: [StageStates."POSITION" ("Action") StageStates."MOVE" ("Action") StageStates."MOVE" ("Action") StageStates."MOVE" ("Action") StageStates."MVR" ("Action") StageStates."MVR" ("Action")] -> w679
              tunnel: w678 -> [_ w696 _ _ _ _]
              tunnel: w677 -> [_ _ w700 _ _ _]
              tunnel: w676 -> [_ _ _ w704 _ _]
              tunnel: [enum16{"MOVE", "MVR"}."MVR" ("MOVE/MVR") enum16{"MOVE", "MVR"}."MOVE" ("MOVE/MVR") enum16{"MOVE", "MVR"}."MOVE" ("MOVE/MVR") enum16{"MOVE", "MVR"}."MOVE" ("MOVE/MVR") enum16{"MOVE", "MVR"}."MVR" ("MOVE/MVR") enum16{"MOVE", "MVR"}."MVR" ("MOVE/MVR")] -> w675
              frame Default {
              }
              frame "MM 1" {
              }
              frame "MM 2" {
              }
              frame "MM 3" {
              }
              frame "Up M227" {
              }
              frame "Down M227" {
                n337 = Negate(x=w714) -> (-x=w713:dbl)
              }
            }
            n338 = Build Array(w680, w680, w680) -> (w682:dbl[])
          }
          frame "Sample Stage XY - M686" {
            n339 = call "M686_Ctrl_Index.vi"("NewVal"=w728, "OldVal"=w729) -> ("M686 - out"=w726:T9, "Control out"=w727:refnum<vi>)  [unwired: 8 in]
            n340 = Unbundle By Name(w726) -> ("Step Size (um)"=w725:dbl, "X"=w724:dbl, "Y"=w723:dbl)
            n341 = property class="Ctl"(reference=w727) -> ("Label.Text"=w716:string)  [unwired: 1 in, 2 out]
            n342 = case shown="\"Left Button\"" w716 {
              tunnel: w725 -> [_ _ w741 w746 w754 w759 _]
              tunnel: w724 -> [_ _ _ _ _ _ w766]
              tunnel: w723 -> [_ _ _ _ _ _ w765]
              tunnel: [StageStates."POSITION" ("Action") StageStates."MOVE" ("Action") StageStates."MVR" ("Action") StageStates."MVR" ("Action") StageStates."MVR" ("Action") StageStates."MVR" ("Action") StageStates."MOVE" ("Action")] -> w721
              tunnel: [enum16{"MOVE", "MVR"}."MVR" ("MOVE/MVR") enum16{"MOVE", "MVR"}."MOVE" ("MOVE/MVR") enum16{"MOVE", "MVR"}."MVR" ("MOVE/MVR") enum16{"MOVE", "MVR"}."MVR" ("MOVE/MVR") enum16{"MOVE", "MVR"}."MVR" ("MOVE/MVR") enum16{"MOVE", "MVR"}."MVR" ("MOVE/MVR") enum16{"MOVE", "MVR"}."MOVE" ("MOVE/MVR")] -> w720
              tunnel: [w731 dbl[] [12.5, 12.5] w739 w747 w755 w761 w767] -> w718
              tunnel: [bool[] [FALSE, FALSE] bool[] [TRUE, TRUE] bool[] [TRUE, TRUE] bool[] [TRUE, TRUE] bool[] [TRUE, TRUE] bool[] [TRUE, TRUE] bool[] [TRUE, TRUE]] -> w717
              frame Default {
                w732 = 0.0 ("Step Size (mm)")
                n343 = Build Array(w732, w732) -> (w731:dbl[])
              }
              frame "Home Button" {
              }
              frame "Right Button" {
                n344 = Build Array(w741, 0.0 ("element")) -> (w739:dbl[])
              }
              frame "Left Button" {
                n345 = Negate(x=w746) -> (-x=w745:dbl)
                n346 = Build Array(w745, 0.0 ("element")) -> (w747:dbl[])
              }
              frame "Up Button" {
                n347 = Negate(x=w754) -> (-x=w753:dbl)
                n348 = Build Array(0.0 ("element"), w753) -> (w755:dbl[])
              }
              frame "Down Button" {
                n349 = Build Array(0.0 ("element"), w759) -> (w761:dbl[])
              }
              frame "X", "Y" {
                n350 = Build Array(w766, w765) -> (w767:dbl[])
              }
            }
          }
        }
        n351 = case shown="Default" w462 {
          frame Default {
          }
          frame "Upper Objective Z - N664" {
            n352 = while {
              i -> [w776]
              stop <- w772 stop-if-true
              n353 = call "Stage_position_ae.vi"("StageID"="N664", "Enum"=enum16{"WRITE", "READ", "HOME", "SAVE HOME"}."READ") -> ("Status Out"=w773:bool, "Position Out"=w783:dbl[])  [unwired: 8 in]
              n354 = Greater?(x=w776, y=200) -> (0:w775:bool)
              n355 = And(x=w773, y=w775) -> (x .and. y?=w772:bool)
              n356 = Wait (ms)(milliseconds to wait=u32 1) -> ()  [unwired: 1 out]
              n357 = Index Array(array=w783, index=0) -> (element=w782:dbl)
              n358 = Select(t=u32 16777215, s=w772, f=u32 6618880) -> (s? t:f=w777:u32)
              n359 = property on="Position (mm)" class="DigNum (strict)"("Value"=w782, "NumText.BG Color"=w777) -> ()  [unwired: 2 in, 2 out]
            }
          }
          frame "Cavity Translation Z - ASI" {
            n360 = while {
              shift-right: [w790] -> _
              shift-left: TRUE ("Status Out") -> [w795]
              stop <- w794 stop-if-true
              n361 = call "Stage_position_ae.vi"("StageID"="ASI", "Enum"=enum16{"WRITE", "READ", "HOME", "SAVE HOME"}."READ") -> ("Status Out"=w790:bool, "Position Out"=w798:dbl[])  [unwired: 8 in]
              n362 = Greater?(x=w790, y=w795) -> (0:w794:bool)
              n363 = Wait (ms)(milliseconds to wait=u32 1) -> ()  [unwired: 1 out]
              n364 = Index Array(array=w798, index=0) -> (element=w788:dbl)
              n365 = Divide(x=w788, y=10.0) -> (x/y=w789:dbl)
              n366 = Select(t=u32 16777215, s=w790, f=u32 6618880) -> (s? t:f=w791:u32)
              n367 = property on="Z (um)" class="DigNum (strict)"("Value"=w789, "NumText.BG Color"=w791) -> ()  [unwired: 2 in, 2 out]
            }
          }
        }
        n368 = control-ref of="Abort AllStage"() -> (w453:refnum<vi>)
        n369 = call "AllStage_Limits_Array.vi"("Step(um)/Position(units)"=w460, "Axis"=w459, "Stage ID"=w461, "MOVE/MVR"=w458) -> ("Positions"=w456:dbl[], "Boolean Array"=w455:bool[], "Stage ID"=w457:string)  [unwired: 4 in, 1 out]
        n370 = call "AE_AllStages_Action V2.vi"("Velocity"=w454, "Abort"=w453, "Positions"=w456, "Axis"=w455, "Stage ID"=w457, "Action"=w452) -> ()  [unwired: 3 in, 3 out]
      }
      event "Stages": Value Change {
        n371 = event-data() -> ("NewVal"=w812:T11)  [unwired: 1 in, 2 out]
        n372 = Unbundle By Name(w812) -> ("M686"=w800:bool, "P841"=w810:bool, "ASI"=w808:bool, "N664"=w806:bool, "P612"=w804:bool, "M227"=w802:bool)
        n373 = call "All_Stages_Aloha.vi"("Aloha"=w800, "Stage ID"="M686") -> ()  [unwired: 9 in, 1 out]
        n374 = call "All_Stages_Aloha.vi"("Aloha"=w810, "Stage ID"="P841") -> ()  [unwired: 9 in, 1 out]
        n375 = call "All_Stages_Aloha.vi"("Aloha"=w808, "Stage ID"="ASI") -> ()  [unwired: 9 in, 1 out]
        n376 = call "All_Stages_Aloha.vi"("Aloha"=w806, "Stage ID"="N664") -> ()  [unwired: 9 in, 1 out]
        n377 = call "All_Stages_Aloha.vi"("Aloha"=w804, "Stage ID"="P612") -> ()  [unwired: 9 in, 1 out]
        n378 = call "All_Stages_Aloha.vi"("Aloha"=w802, "Stage ID"="M227") -> ()  [unwired: 9 in, 1 out]
      }
      event "SLM", "Timing", "DM", "Camera", "Focus Lock", "Stage Monitor": Value Change {
        n379 = event-data() -> ("CtlRef"=w816:refnum<vi>, "NewVal"=w813:bool)  [unwired: 1 in, 1 out]
        n380 = property class="Bool (strict)"(reference=w816) -> ("Label.Text"=w815:string)  [unwired: 1 in, 2 out]
        n381 = case shown="\"DM\"" w815 {
          tunnel: w813 -> [w817 w831 w845 w859 w872 w889]
          frame "SLM", Default {
            n382 = case shown="True" w817 {
              frame False {
                n383 = To Variant(anything=TRUE) -> (Variant=w823:variant)
                n384 = call "SLM AE.vi"("Action"=enum16{"READ", "WRITE"}."READ") -> ("SLM Ref Out"=w824:refnum<vi>)  [unwired: 10 in]
                n385 = invoke class="VI" method="Ctrl Val.Set"(reference=w824, "Control Name"="Exit", "Value"=w823) -> (reference out=w820:refnum<vi>, error out=w819:errorcluster)  [unwired: 2 in, 3 out]
                n386 = invoke on="Hamamatsu LCOS" class="SubPnl" method="Remove VI"(error in=w819) -> (error out=w818:errorcluster)  [unwired: 2 in, 2 out]
                n387 = Close Reference(reference=w820, error in (no error)=w818) -> ()  [unwired: 1 out]
              }
              frame True {
                n388 = Open VI Reference(vi path=path "C:/Users/ED STED/Documents/Test Control Software/Host VIs/SLM_V2/SLM Control.vi") -> (vi reference=w829:refnum<vi>)  [unwired: 5 in, 1 out]
                n389 = invoke class="VI" method="Run VI"(reference=w829, "Wait until done"=FALSE ("Wait Until Done")) -> (reference out=w826:refnum<vi>)  [unwired: 3 in, 4 out]
                n390 = invoke on="Hamamatsu LCOS" class="SubPanel" method="Insert VI"("VI Ref"=w826) -> ()  [unwired: 3 in, 4 out]
                n391 = call "SLM AE.vi"("Action"=enum16{"READ", "WRITE"}."WRITE", "SLM Ref In"=w826) -> ()  [unwired: 9 in, 1 out]
              }
            }
          }
          frame "DM" {
            n392 = case shown="True" w831 {
              frame False {
                n393 = call "DM_Ref_AE.vi"("Action"=enum16{"READ", "WRITE"}."READ") -> ("DM Ref Out"=w838:refnum<vi>)  [unwired: 10 in]
                n394 = To Variant(anything=TRUE) -> (Variant=w837:variant)
                n395 = invoke class="VI" method="Ctrl Val.Set"(reference=w838, "Control Name"="Exit", "Value"=w837) -> (reference out=w834:refnum<vi>, error out=w833:errorcluster)  [unwired: 2 in, 3 out]
                n396 = invoke on="BM Multi" class="SubPnl" method="Remove VI"(error in=w833) -> (error out=w832:errorcluster)  [unwired: 2 in, 2 out]
                n397 = Close Reference(reference=w834, error in (no error)=w832) -> ()  [unwired: 1 out]
              }
              frame True {
                n398 = Open VI Reference(vi path=path "C:/Users/ED STED/Documents/Test Control Software/Host VIs/DM_Dual_V2/Dual_DM_Control_Main_V5.vi") -> (vi reference=w843:refnum<vi>)  [unwired: 5 in, 1 out]
                n399 = invoke class="VI" method="Run VI"(reference=w843, "Wait until done"=FALSE ("Wait Until Done")) -> (reference out=w840:refnum<vi>)  [unwired: 3 in, 4 out]
                n400 = invoke on="BM Multi" class="SubPanel" method="Insert VI"("VI Ref"=w840) -> ()  [unwired: 3 in, 4 out]
                n401 = call "DM_Ref_AE.vi"("Action"=enum16{"READ", "WRITE"}."WRITE", "DM Ref In"=w840) -> ()  [unwired: 9 in, 1 out]
              }
            }
          }
          frame "Timing" {
            n402 = case shown="True" w845 {
              frame False {
                n403 = To Variant(anything=TRUE) -> (Variant=w850:variant)
                n404 = call "GateDelay AE.vi"("Action"=enum16{"READ", "WRITE"}."READ") -> ("Gate Delay Ref Out"=w851:refnum<vi>)  [unwired: 10 in]
                n405 = invoke class="VI" method="Ctrl Val.Set"(reference=w851, "Control Name"="Exit", "Value"=w850) -> (reference out=w846:refnum<vi>, error out=w847:errorcluster)  [unwired: 2 in, 3 out]
                n406 = invoke on="Timing" class="SubPnl" method="Remove VI"(error in=w847) -> (error out=w853:errorcluster)  [unwired: 2 in, 2 out]
                n407 = Close Reference(reference=w846, error in (no error)=w853) -> ()  [unwired: 1 out]
              }
              frame True {
                n408 = Open VI Reference(vi path=path "C:/Users/ED STED/Documents/Test Control Software/Host VIs/Time Delay/GateDelay_Control_V2.vi") -> (vi reference=w856:refnum<vi>)  [unwired: 5 in, 1 out]
                n409 = invoke class="VI" method="Run VI"(reference=w856, "Wait until done"=FALSE ("Wait Until Done")) -> (reference out=w855:refnum<vi>)  [unwired: 3 in, 4 out]
                n410 = invoke on="Timing" class="SubPanel" method="Insert VI"("VI Ref"=w855) -> ()  [unwired: 3 in, 4 out]
                n411 = call "GateDelay AE.vi"("Action"=enum16{"READ", "WRITE"}."WRITE", "Gate Delay Ref In"=w855) -> ()  [unwired: 9 in, 1 out]
              }
            }
          }
          frame "Camera" {
            n412 = case shown="False" w859 {
              frame False {
                n413 = To Variant(anything=TRUE) -> (Variant=w860:variant)
                n414 = call "Camera_Ref_HX.vi"("Action"=enum16{"READ", "WRITE"}."READ") -> ("Alignment Ref Out"=w864:refnum<vi>)  [unwired: 10 in]
                n415 = invoke class="VI" method="Ctrl Val.Set"(reference=w864, "Control Name"="Exit", "Value"=w860) -> (reference out=w863:refnum<vi>)  [unwired: 2 in, 4 out]
                n416 = invoke on="Tool Box" class="SubPnl" method="Remove VI"() -> (error out=w865:errorcluster)  [unwired: 3 in, 2 out]
                n417 = Close Reference(reference=w863, error in (no error)=w865) -> ()  [unwired: 1 out]
              }
              frame True {
                n418 = Open VI Reference(vi path=path "C:/Users/ED STED/Documents/Test Control Software/Host VIs/Camera/uEye_Control_V1.vi") -> (vi reference=w869:refnum<vi>)  [unwired: 5 in, 1 out]
                n419 = invoke class="VI" method="Run VI"(reference=w869, "Wait until done"=FALSE ("Wait Until Done")) -> (reference out=w868:refnum<vi>)  [unwired: 3 in, 4 out]
                n420 = invoke on="Tool Box" class="SubPnl" method="Insert VI"("VI Ref"=w868) -> ()  [unwired: 3 in, 4 out]
                n421 = call "Camera_Ref_HX.vi"("Action"=enum16{"READ", "WRITE"}."WRITE", "Alignment Ref In"=w868) -> ()  [unwired: 9 in, 1 out]
              }
            }
          }
          frame "Focus Lock" {
            n422 = case shown="True" w872 {
              frame False {
                n423 = call "Lock Control AE.vi"("Action"=Standard_Action_for_Focus_Lock."Read") -> ("Lock Control  out"=w875:T38)  [unwired: 1 in]
                n424 = Bundle By Name(cluster=w875, "EXIT"=TRUE) -> (w873:T38)
                n425 = call "FocusLock_Ref_HX.vi"("Action"=enum16{"READ", "WRITE"}."READ") -> ("FocusLock Ref Out"=w881:refnum<vi>)  [unwired: 10 in]
                n426 = To Variant(anything=w873) -> (Variant=w879:variant)
                n427 = invoke class="VI" method="Ctrl Val.Set"(reference=w881, "Control Name"="Lock Control", "Value"=w879) -> (reference out=w880:refnum<vi>, error out=w878:errorcluster)  [unwired: 2 in, 3 out]
                n428 = invoke on="Focus Lock\nFocus Lock Panel" class="SubPnl" method="Remove VI"(error in=w878) -> (error out=w882:errorcluster)  [unwired: 2 in, 2 out]
                n429 = Close Reference(reference=w880, error in (no error)=w882) -> ()  [unwired: 1 out]
              }
              frame True {
                n430 = Open VI Reference(vi path=path "C:/Users/ED STED/Documents/Test Control Software/Host VIs/Focus Lock/FocusLock Control v2.vi") -> (vi reference=w886:refnum<vi>)  [unwired: 5 in, 1 out]
                n431 = invoke class="VI" method="Run VI"(reference=w886, "Wait until done"=FALSE ("Wait Until Done")) -> (reference out=w885:refnum<vi>)  [unwired: 3 in, 4 out]
                n432 = invoke on="Focus Lock\nFocus Lock Panel" class="SubPnl" method="Insert VI"("VI Ref"=w885) -> ()  [unwired: 3 in, 4 out]
                n433 = call "FocusLock_Ref_HX.vi"("Action"=enum16{"READ", "WRITE"}."WRITE", "FocusLock Ref In"=w885) -> ()  [unwired: 9 in, 1 out]
              }
            }
          }
          frame "Stage Monitor" {
            n434 = case shown="True" w889 {
              frame False {
                n435 = call "StageMonitor_Ref_HX.vi"("Action"=enum16{"READ", "WRITE"}."READ") -> ("StageMonitor Ref Out"=w892:refnum<vi>)  [unwired: 10 in]
                n436 = To Variant(anything=TRUE) -> (Variant=w895:variant)
                n437 = invoke class="VI" method="Ctrl Val.Set"(reference=w892, "Control Name"="Exit", "Value"=w895) -> (reference out=w896:refnum<vi>, error out=w894:errorcluster)  [unwired: 2 in, 3 out]
                n438 = invoke on="Tool Box 2" class="SubPnl" method="Remove VI"(error in=w894) -> (error out=w897:errorcluster)  [unwired: 2 in, 2 out]
                n439 = Close Reference(reference=w896, error in (no error)=w897) -> ()  [unwired: 1 out]
              }
              frame True {
                n440 = Open VI Reference(vi path=path "C:/Users/ED STED/Documents/Test Control Software/Host VIs/Stages/Stage Monitor/Stage Monitor.vi") -> (vi reference=w900:refnum<vi>)  [unwired: 5 in, 1 out]
                n441 = invoke class="VI" method="Run VI"(reference=w900, "Wait until done"=FALSE ("Wait Until Done")) -> (reference out=w899:refnum<vi>)  [unwired: 3 in, 4 out]
                n442 = invoke on="Tool Box 2" class="SubPnl" method="Insert VI"("VI Ref"=w899) -> ()  [unwired: 3 in, 4 out]
                n443 = call "StageMonitor_Ref_HX.vi"("Action"=enum16{"READ", "WRITE"}."WRITE", "StageMonitor Ref In"=w899) -> ()  [unwired: 9 in, 1 out]
              }
            }
          }
        }
      }
      event Value Change {
        n444 = event-data() -> ("CtlRef"=w908:refnum<vi>, "OldVal"=w906:variant, "NewVal"=w905:variant)  [unwired: 1 in]
        n445 = property class="Clust"(reference=w908) -> ("Label.Text"=w907:string)  [unwired: 1 in, 2 out]
        n446 = call "Graph Ref AE.vi"("Action"=enum16{"READ", "WRITE"}."READ") -> ("Graph Ref Out"=w903:refnum<vi>[])  [unwired: 10 in]
        n447 = case shown="\"Graph Tools\"" w907 {
          tunnel: w906 -> [_ w915 w971]
          tunnel: w905 -> [_ w916 w970]
          tunnel: w903 -> [_ w910 w963]
          frame Default {
          }
          frame "Display Controls" {
            n448 = call "Display_Controls_Ctrl_Index.vi"("OldVal"=w915, "NewVal"=w916) -> ("Control Ref OUT"=w914:refnum<vi>, "Display Controls Out"=w912:T3)  [unwired: 12 in]
            n449 = property class="Ctl"(reference=w914) -> ("Label.Text"=w913:string)  [unwired: 1 in, 2 out]
            n450 = Unbundle By Name(w912) -> ("Single Screen"=w911:bool)
            n451 = case shown="\"Single Screen\", Default" w913 {
              tunnel: w911 -> [w924 _ _]
              tunnel: w910 -> [_ w949 w956]
              frame "Single Screen", Default {
                n452 = property class="App"() -> ("Disp.AllMonitors"=w923:T39)  [unwired: 2 in, 2 out]
                n453 = Index Array(array=w923, index #1=2 ("index"), index #2=0 ("index")) -> (element #1=w920:T40, element #2=w919:T40)
                n454 = control-ref of="This VI"() -> (w918:refnum<vi>)
                n455 = case shown="False" w924 {
                  tunnel: w920 -> [w928 _]
                  tunnel: w919 -> [w927 w939]
                  tunnel: w918 -> [w926 w937]
                  tunnel: T26 {"Left"=0, "Top"=0, "Right"=0, "Bottom"=0} ("Front Panel Window:Window Bounds") -> [w925 w938]
                  frame False {
                    w933 = i16 0
                    n456 = Unbundle By Name(w927) -> ("Bounds.Left"=w930:i16, "Bounds.Bottom"=w931:i16, "Bounds.Top"=w932:i16)
                    n457 = Unbundle By Name(w928) -> ("Bounds.Right"=w929:i16)
                    n458 = Subtract(x=w929, y=w930) -> (x-y=w934:i16)
                    n459 = Subtract(x=w931, y=w932) -> (x-y=w935:i16)
                    n460 = Bundle By Name(cluster=w925, "Left"=w933, "Top"=w933, "Right"=w934, "Bottom"=w935) -> (w936:T26)
                    n461 = property class="VI"(reference=w926, "Front Panel.WinBounds"=w936) -> ()  [unwired: 1 in, 2 out]
                  }
                  frame True {
                    w942 = i16 0
                    n462 = Unbundle By Name(w939) -> ("Bounds.Right"=w945:i16, "Bounds.Bottom"=w944:i16, "Bounds.Top"=w943:i16)
                    n463 = Subtract(x=w944, y=w943) -> (x-y=w941:i16)
                    n464 = Bundle By Name(cluster=w938, "Left"=w942, "Top"=w942, "Right"=w945, "Bottom"=w941) -> (w940:T26)
                    n465 = property class="VI"(reference=w937, "Front Panel.WinBounds"=w940) -> (reference out=w947:refnum<vi>)  [unwired: 1 in, 1 out]
                    n466 = property class="VI"(reference=w947, "FP.State"=T27."Maximized" ("Front Panel Window:State")) -> ()  [unwired: 1 in, 2 out]
                  }
                }
              }
              frame "Add Display" {
                w950 = u16 0 items=["Read", "Write"] ("Action")
                w954 = u16 1 items=["Read", "Write"] ("Action")
                n467 = property on="Add Display" class="Bool (strict)"("Value"=FALSE) -> ()  [unwired: 2 in, 2 out]
                n468 = call "Arange_Displays_V2.vi"("Action"=w950) -> ("Number of Channels OUT"=w951:i32)  [unwired: 14 in]
                n469 = Increment(x=w951) -> (x+1=w953:i32)
                n470 = call "Arange_Displays_V2.vi"("Display References"=w949, "Action"=w954, "Number of Channels"=w953, "Aspect Ratio (h/w)"=1.0) -> ()  [unwired: 11 in, 1 out]
              }
              frame "Remove Display" {
                w957 = u16 0 items=["Read", "Write"] ("Action")
                w961 = u16 1 items=["Read", "Write"] ("Action")
                n471 = call "Arange_Displays_V2.vi"("Action"=w957) -> ("Number of Channels OUT"=w958:i32)  [unwired: 14 in]
                n472 = Decrement(x=w958) -> (x-1=w960:i32)
                n473 = call "Arange_Displays_V2.vi"("Display References"=w956, "Action"=w961, "Number of Channels"=w960, "Aspect Ratio (h/w)"=1.0) -> ()  [unwired: 11 in, 1 out]
                n474 = property on="Remove Display" class="Bool (strict)"("Value"=FALSE) -> ()  [unwired: 2 in, 2 out]
              }
            }
          }
          frame "Graph Tools" {
            n475 = call "Graph_Controls_Ctrl_Index.vi"("OldVal"=w971, "NewVal"=w970) -> ("Control Ref OUT"=w969:refnum<vi>, "Graph Tools Out"=w968:T4)  [unwired: 12 in]
            n476 = property class="Ctl"(reference=w969) -> (reference out=w965:refnum<vi>, "Label.Text"=w964:string)  [unwired: 1 in, 1 out]
            n477 = Unbundle By Name(w968) -> ("Show Cursor"=w967:bool, "Auto Scale"=w966:bool, "Color Map"=w962:T41)
            n478 = case shown="\"Fit Tool\"" w964 {
              selector: w964 -> [_ _ _ w1042 _ _ _ _]
              tunnel: w967 -> [_ w1011 _ _ _ _ _ _]
              tunnel: w966 -> [_ _ w1031 _ _ _ _ _]
              tunnel: w963 -> [w980 w1010 w1032 w1035 w1072 w1079 w1092 w1100]
              tunnel: w965 -> [_ _ _ _ _ _ _ _]
              tunnel: w964 -> [_ _ _ w1037 _ _ _ _]
              tunnel: w962 -> [w983 _ _ _ _ _ _ _]
              frame "Apply Color" {
                n479 = control-ref of="This VI"() -> (w982:refnum<vi>)
                n480 = call "GetDisplayClick.vi"("Display REFs In"=w980, "Calling VI REF"=w982) -> ("Display Index"=w981:i32)  [unwired: 13 in]
                n481 = Index Array(array=w980, index=w981) -> (element=w979:refnum<vi>)
                n482 = property class="IntGraph (strict)"(reference=w979) -> (reference out=w975:refnum<vi>, error out=w972:errorcluster, "ZScale.Maximum"=w978:dbl)  [unwired: 1 in]
                n483 = case shown="\"Gray\"" w983 {
                  tunnel: [cluster{dbl, u32}[] [{0.0, 0}, {0.07843137254901933, 131072}, {0.15686274509805287, 196608}, {0.235294117647058, 327680}, {0.3137254901960773, 458752}, {0.39215686274509665, 589824}, {0.47058823529410176, 720896}, {0.5490196078431353, 851971}, {0.6274509803921546, 983043}, {0.705882352941174, 1114115}, {0.7843137254902075, 1245187}, {0.8627450980392268, 1376259}, {0.941176470588232, 1507331}, {1.0196078431372513, 1638403}, {1.0980392156862848, 1769475}, {1.1764705882353041, 1769479}, {1.2549019607843093, 2031623}, {1.3333333333333286, 2162695}, {1.4117647058823621, 2293767}, {1.4901960784313673, 2424839}, {1.5686274509803866, 2555911}, {1.647058823529406, 2686983}, {1.7254901960784395, 2818055}, {1.8039215686274588, 2949127}, {1.882352941176464, 3080203}, {1.9607843137254832, 3211275}, {2.0392156862745168, 3342347}, {2.117647058823522, 3473419}, {2.1960784313725554, 3604491}, {2.2745098039215605, 3735563}, {2.352941176470594, 3866635}, {2.431372549019599, 3867403}, {2.5098039215686327, 4129547}, {2.588235294117638, 4260619}, {2.6666666666666714, 4391691}, {2.7450980392156907, 4522763}, {2.823529411764696, 4653839}, {2.901960784313715, 4784911}, {2.9803921568627487, 4915983}, {3.058823529411768, 5178127}, {3.1372549019607874, 5309199}, {3.2156862745097925, 5440271}, {3.294117647058826, 5571343}, {3.3725490196078454, 5702415}, {3.4509803921568647, 5703439}, {3.52941176470587, 5965583}, {3.6078431372549034, 6096655}, {3.6862745098039227, 6227727}, {3.764705882352942, 6358799}, {3.8431372549019756, 6489871}, {3.9215686274509807, 6620943}, {4.0, 6752015}, {4.078431372549019, 6883087}, {4.1568627450980244, 7015183}, {4.235294117647058, 7146255}, {4.313725490196077, 7277327}, {4.392156862745097, 7408399}, {4.470588235294102, 7539471}, {4.549019607843135, 7670543}, {4.627450980392155, 7801615}, {4.705882352941174, 8063759}, {4.784313725490179, 8194831}, {4.862745098039213, 8326927}, {4.941176470588232, 8457999}, {5.019607843137251, 8589075}, {5.098039215686285, 8720147}, {5.17647058823529, 8851219}, {5.254901960784309, 8982291}, {5.333333333333329, 9113363}, {5.411764705882362, 9114387}, {5.490196078431367, 9376531}, {5.568627450980401, 9507603}, {5.647058823529406, 9638675}, {5.7254901960784395, 9769747}, {5.803921568627445, 9901843}, {5.882352941176478, 10032915}, {5.960784313725483, 10163987}, {6.039215686274517, 10229523}, {6.117647058823522, 10295059}, {6.196078431372555, 10427155}, {6.2745098039215605, 10558227}, {6.352941176470594, 10689299}, {6.431372549019599, 10820371}, {6.509803921568633, 10886931}, {6.588235294117638, 10952467}, {6.666666666666671, 11083539}, {6.745098039215691, 11214611}, {6.82352941176471, 11215635}, {6.901960784313715, 11477779}, {6.980392156862749, 11543315}, {7.058823529411768, 11608851}, {7.137254901960787, 11740947}, {7.215686274509821, 11806483}, {7.294117647058826, 11872019}, {7.372549019607845, 12004115}, {7.450980392156865, 12135187}, {7.529411764705898, 12266259}, {7.607843137254903, 12267283}, {7.686274509803923, 12398355}, {7.764705882352942, 12529427}, {7.843137254901947, 12530451}, {7.921568627450981, 12595987}, {8.0, 12530451}, {8.07843137254902, 12793619}, {8.156862745098024, 12794131}, {8.235294117647058, 12794643}, {8.313725490196077, 13056787}, {8.392156862745097, 13057299}, {8.47058823529413, 13057811}, {8.549019607843135, 13188883}, {8.627450980392155, 13320979}, {8.705882352941174, 13386515}, {8.784313725490179, 13452563}, {8.862745098039213, 13584147}, {8.941176470588232, 13584659}, {9.019607843137251, 13585171}, {9.098039215686256, 13585683}, {9.17647058823529, 13717267}, {9.254901960784323, 13848339}, {9.333333333333329, 13849363}, {9.411764705882362, 13849875}, {9.490196078431367, 13850387}, {9.5686274509804, 13981459}, {9.647058823529406, 14113555}, {9.72549019607844, 14114067}, {9.803921568627445, 14114579}, {9.882352941176478, 14115091}, {9.960784313725483, 14246675}, {10.039215686274517, 14377747}, {10.117647058823522, 14378771}, {10.196078431372555, 14379283}, {10.27450980392156, 14379539}, {10.352941176470594, 14379795}, {10.4313725490196, 14380819}, {10.509803921568633, 14511891}, {10.588235294117638, 14643987}, {10.666666666666671, 14644503}, {10.745098039215677, 14645015}, {10.82352941176471, 14645527}, {10.901960784313744, 14646039}, {10.980392156862749, 14646551}, {11.058823529411768, 14778135}, {11.137254901960787, 14909207}, {11.215686274509821, 14910231}, {11.294117647058826, 14910747}, {11.372549019607845, 14911259}, {11.450980392156865, 14911771}, {11.52941176470587, 14912283}, {11.607843137254903, 14912797}, {11.686274509803923, 15044383}, {11.764705882352942, 15175455}, {11.843137254901947, 15175967}, {11.92156862745098, 15176479}, {12.0, 15176991}, {12.07843137254902, 15177507}, {12.156862745098053, 15178019}, {12.235294117647058, 15178531}, {12.313725490196092, 15310115}, {12.392156862745097, 15441701}, {12.47058823529413, 15441959}, {12.549019607843135, 15442215}, {12.627450980392155, 15442727}, {12.705882352941174, 15443243}, {12.784313725490179, 15443755}, {12.862745098039213, 15444269}, {12.941176470588246, 15444783}, {13.019607843137251, 15444783}, {13.098039215686285, 15576367}, {13.17647058823529, 15707953}, {13.25490196078431, 15708467}, {13.333333333333329, 15708979}, {13.411764705882362, 15708981}, {13.490196078431367, 15708983}, {13.568627450980387, 15710011}, {13.647058823529406, 15710523}, {13.725490196078411, 15711037}, {13.803921568627459, 15711039}, {13.882352941176464, 15711553}, {13.960784313725512, 15843139}, {14.039215686274517, 15974213}, {14.117647058823522, 15974215}, {14.196078431372541, 15974217}, {14.27450980392156, 15974219}, {14.352941176470594, 15975755}, {14.431372549019613, 15976271}, {14.509803921568633, 15976785}, {14.588235294117666, 15977299}, {14.666666666666671, 15977301}, {14.745098039215677, 15977815}, {14.82352941176471, 15978327}, {14.901960784313744, 15978331}, {14.980392156862749, 16109917}, {15.058823529411768, 16241503}, {15.137254901960787, 16241505}, {15.215686274509792, 16242019}, {15.294117647058826, 16242535}, {15.372549019607845, 16242537}, {15.450980392156865, 16242539}, {15.529411764705898, 16243563}, {15.607843137254903, 16243567}, {15.686274509803908, 16244081}, {15.764705882352942, 16244595}, {15.843137254901947, 16244599}, {15.92156862745098, 16244601}, {16.0, 16244603}, {16.07843137254902, 16245627}, {16.156862745098024, 16245631}, {16.235294117647058, 16245633}, {16.313725490196077, 16246147}, {16.392156862745097, 16246663}, {16.47058823529413, 16377735}, {16.549019607843135, 16508811}, {16.62745098039217, 16508815}, {16.705882352941174, 16509839}, {16.78431372549018, 16509843}, {16.862745098039213, 16509845}, {16.941176470588232, 16509847}, {17.01960784313725, 16510361}, {17.098039215686256, 16510875}, {17.17647058823529, 16510879}, {17.25490196078431, 16510881}, {17.33333333333333, 16510883}, {17.411764705882362, 16511399}, {17.49019607843138, 16511911}, {17.568627450980387, 16511915}, {17.647058823529406, 16511917}, {17.72549019607844, 16511919}, {17.80392156862746, 16511923}, {17.882352941176464, 16512437}, {17.960784313725483, 16512951}, {18.03921568627449, 16512955}, {18.117647058823522, 16512957}, {18.19607843137254, 16512959}, {18.27450980392156, 16512961}, {18.352941176470594, 16512963}, {18.431372549019613, 16512967}, {18.509803921568633, 16513481}, {18.588235294117638, 16513995}, {18.66666666666667, 16513999}, {18.74509803921569, 16514001}, {18.82352941176471, 16514003}, {18.901960784313744, 16514005}, {18.98039215686275, 16514007}, {19.058823529411754, 16514011}, {19.137254901960787, 16514013}, {19.215686274509792, 16514015}, {19.294117647058826, 16514019}, {19.372549019607845, 16514021}, {19.450980392156865, 16514023}, {19.52941176470587, 16514027}, {19.607843137254918, 16514029}, {19.686274509803923, 16514031}, {19.764705882352942, 16514035}, {19.843137254901947, 16514037}, {19.921568627450995, 16514039}, {20.0, 16514043}] ("Z Scale.Marker Values[]") cluster{dbl, u32}[] [{0.0, 0}, {85.0, 16711680}, {108.0, 16729344}, {127.0, 16744192}, {132.0, 16747520}, {140.0, 16753920}, {157.0, 16766720}, {170.0, 16776960}, {245.0, 16777184}, {250.0, 16777200}, {255.0, 16777215}] ("Z Scale.Marker Values[]") cluster{dbl, u32}[] [{0.0, 0}, {255.0, 16777215}] ("Z Scale.Marker Values[]") cluster{dbl, u32}[] [{0.0, 0}, {255.0, 16711680}] ("Z Scale.Marker Values[]") cluster{dbl, u32}[] [{0.0, 0}, {255.0, 65280}] ("Z Scale.Marker Values[]") cluster{dbl, u32}[] [{0.0, 0}, {255.0, 255}] ("Z Scale.Marker Values[]") cluster{dbl, u32}[] [{0.0, 0}, {255.0, 65535}] ("Z Scale.Marker Values[]") cluster{dbl, u32}[] [{0.0, 0}, {255.0, 16711935}] ("Z Scale.Marker Values[]") cluster{dbl, u32}[] [{0.0, 0}, {255.0, 16776960}] ("Z Scale.Marker Values[]") cluster{dbl, u32}[] [{0.0, 0}, {170.0, 16711680}, {245.0, 16777184}, {250.0, 16777200}, {255.0, 16448250}] ("Z Scale.Marker Values[]") cluster{dbl, u32}[] [{0.0, 0}, {170.0, 65280}, {245.0, 16777184}, {250.0, 16777200}, {255.0, 16448250}] ("Z Scale.Marker Values[]") cluster{dbl, u32}[] [{0.0, 0}, {170.0, 255}, {245.0, 16777184}, {250.0, 16777200}, {255.0, 16448250}] ("Z Scale.Marker Values[]") cluster{dbl, u32}[] [{0.0, 0}, {1.0, 131072}, {2.0, 196608}, {3.0, 327680}, {4.0, 458752}, {5.0, 589824}, {6.0, 720896}, {7.0, 851971}, {8.0, 983043}, {9.0, 1114115}, {10.0, 1245187}, {11.0, 1376259}, {12.0, 1507331}, {13.0, 1638403}, {14.0, 1769475}, {15.0, 1769479}, {16.0, 2031623}, {17.0, 2162695}, {18.0, 2293767}, {19.0, 2424839}, {20.0, 2555911}, {21.0, 2686983}, {22.0, 2818055}, {23.0, 2949127}, {24.0, 3080203}, {25.0, 3211275}, {26.0, 3342347}, {27.0, 3473419}, {28.0, 3604491}, {29.0, 3735563}, {30.0, 3866635}, {31.0, 3867403}, {32.0, 4129547}, {33.0, 4260619}, {34.0, 4391691}, {35.0, 4522763}, {36.0, 4653839}, {37.0, 4784911}, {38.0, 4915983}, {39.0, 5178127}, {40.0, 5309199}, {41.0, 5440271}, {42.0, 5571343}, {43.0, 5702415}, {44.0, 5703439}, {45.0, 5965583}, {46.0, 6096655}, {47.0, 6227727}, {48.0, 6358799}, {49.0, 6489871}, {50.0, 6620943}, {51.0, 6752015}, {52.0, 6883087}, {53.0, 7015183}, {54.0, 7146255}, {55.0, 7277327}, {56.0, 7408399}, {57.0, 7539471}, {58.0, 7670543}, {59.0, 7801615}, {60.0, 8063759}, {61.0, 8194831}, {62.0, 8326927}, {63.0, 8457999}, {64.0, 8589075}, {65.0, 8720147}, {66.0, 8851219}, {67.0, 8982291}, {68.0, 9113363}, {69.0, 9114387}, {70.0, 9376531}, {71.0, 9507603}, {72.0, 9638675}, {73.0, 9769747}, {74.0, 9901843}, {75.0, 10032915}, {76.0, 10163987}, {77.0, 10229523}, {78.0, 10295059}, {79.0, 10427155}, {80.0, 10558227}, {81.0, 10689299}, {82.0, 10820371}, {83.0, 10886931}, {84.0, 10952467}, {85.0, 11083539}, {86.0, 11214611}, {87.0, 11215635}, {88.0, 11477779}, {89.0, 11543315}, {90.0, 11608851}, {91.0, 11740947}, {92.0, 11806483}, {93.0, 11872019}, {94.0, 12004115}, {95.0, 12135187}, {96.0, 12266259}, {97.0, 12267283}, {98.0, 12398355}, {99.0, 12529427}, {100.0, 12530451}, {101.0, 12595987}, {102.0, 12530451}, {103.0, 12793619}, {104.0, 12794131}, {105.0, 12794643}, {106.0, 13056787}, {107.0, 13057299}, {108.0, 13057811}, {109.0, 13188883}, {110.0, 13320979}, {111.0, 13386515}, {112.0, 13452563}, {113.0, 13584147}, {114.0, 13584659}, {115.0, 13585171}, {116.0, 13585683}, {117.0, 13717267}, {118.0, 13848339}, {119.0, 13849363}, {120.0, 13849875}, {121.0, 13850387}, {122.0, 13981459}, {123.0, 14113555}, {124.0, 14114067}, {125.0, 14114579}, {126.0, 14115091}, {127.0, 14246675}, {128.0, 14377747}, {129.0, 14378771}, {130.0, 14379283}, {131.0, 14379539}, {132.0, 14379795}, {133.0, 14380819}, {134.0, 14511891}, {135.0, 14643987}, {136.0, 14644503}, {137.0, 14645015}, {138.0, 14645527}, {139.0, 14646039}, {140.0, 14646551}, {141.0, 14778135}, {142.0, 14909207}, {143.0, 14910231}, {144.0, 14910747}, {145.0, 14911259}, {146.0, 14911771}, {147.0, 14912283}, {148.0, 14912797}, {149.0, 15044383}, {150.0, 15175455}, {151.0, 15175967}, {152.0, 15176479}, {153.0, 15176991}, {154.0, 15177507}, {155.0, 15178019}, {156.0, 15178531}, {157.0, 15310115}, {158.0, 15441701}, {159.0, 15441959}, {160.0, 15442215}, {161.0, 15442727}, {162.0, 15443243}, {163.0, 15443755}, {164.0, 15444269}, {165.0, 15444783}, {166.0, 15444783}, {167.0, 15576367}, {168.0, 15707953}, {169.0, 15708467}, {170.0, 15708979}, {171.0, 15708981}, {172.0, 15708983}, {173.0, 15710011}, {174.0, 15710523}, {175.0, 15711037}, {176.0, 15711039}, {177.0, 15711553}, {178.0, 15843139}, {179.0, 15974213}, {180.0, 15974215}, {181.0, 15974217}, {182.0, 15974219}, {183.0, 15975755}, {184.0, 15976271}, {185.0, 15976785}, {186.0, 15977299}, {187.0, 15977301}, {188.0, 15977815}, {189.0, 15978327}, {190.0, 15978331}, {191.0, 16109917}, {192.0, 16241503}, {193.0, 16241505}, {194.0, 16242019}, {195.0, 16242535}, {196.0, 16242537}, {197.0, 16242539}, {198.0, 16243563}, {199.0, 16243567}, {200.0, 16244081}, {201.0, 16244595}, {202.0, 16244599}, {203.0, 16244601}, {204.0, 16244603}, {205.0, 16245627}, {206.0, 16245631}, {207.0, 16245633}, {208.0, 16246147}, {209.0, 16246663}, {210.0, 16377735}, {211.0, 16508811}, {212.0, 16508815}, {213.0, 16509839}, {214.0, 16509843}, {215.0, 16509845}, {216.0, 16509847}, {217.0, 16510361}, {218.0, 16510875}, {219.0, 16510879}, {220.0, 16510881}, {221.0, 16510883}, {222.0, 16511399}, {223.0, 16511911}, {224.0, 16511915}, {225.0, 16511917}, {226.0, 16511919}, {227.0, 16511923}, {228.0, 16512437}, {229.0, 16512951}, {230.0, 16512955}, {231.0, 16512957}, {232.0, 16512959}, {233.0, 16512961}, {234.0, 16512963}, {235.0, 16512967}, {236.0, 16513481}, {237.0, 16513995}, {238.0, 16513999}, {239.0, 16514001}, {240.0, 16514003}, {241.0, 16514005}, {242.0, 16514007}, {243.0, 16514011}, {244.0, 16514013}, {245.0, 16514015}, {246.0, 16514019}, {247.0, 16514021}, {248.0, 16514023}, {249.0, 16514027}, {250.0, 16514029}, {251.0, 16514031}, {252.0, 16514035}, {253.0, 16514037}, {254.0, 16514039}, {255.0, 16514043}] ("Z Scale.Marker Values[]")] -> w974
                  tunnel: w978 -> [w985 w986 w988 w990 w992 w994 w996 w998 w1000 w1002 w1004 w1006 w1009]
                  tunnel: [w985 w986 w988 w990 w992 w994 w996 w998 w1000 w1002 w1004 w1006 w1009] -> w976
                  frame "System", Default {
                  }
                  frame "Fire" {
                    # "Fire"
                  }
                  frame "Gray" {
                    # "Grayscale"
                  }
                  frame "Red" {
                    # "Red"
                  }
                  frame "Green" {
                    # "Green"
                  }
                  frame "Blue" {
                    # "Blue"
                  }
                  frame "Cyan" {
                    # "Cyan"
                  }
                  frame "Magenta" {
                    # "Magenta"
                  }
                  frame "Yellow" {
                    # "Yellow"
                  }
                  frame "Red-White" {
                    # "Red-White"
                  }
                  frame "Green-White" {
                    # "Green-White"
                  }
                  frame "Blue-White" {
                    # "Blue-White"
                  }
                  frame "Glow" {
                  }
                }
                n484 = property on="Apply Color" class="Bool (strict)"(error in=w972, "Value"=FALSE) -> ()  [unwired: 1 in, 2 out]
                n485 = property class="IntGraph (strict)"(reference=w975, "ZScale.MarkerVals[]"=w974, "ZScale.High Color"=u32 255, "ZScale.Maximum"=w976) -> ()  [unwired: 1 in, 2 out]
              }
              frame "Show Cursor", Default {
                w1014 = 2.0 ("y")
                n486 = Index Array(array=w1010, index=0) -> (element=w1022:refnum<vi>)
                n487 = property class="IntGraph (strict)"(reference=w1022) -> ("Value"=w1021:sgl[][])  [unwired: 1 in, 2 out]
                n488 = Array Size(array=w1021) -> (size(s)=w1020:i32[])
                n489 = To Double Precision Float(number=w1020) -> (double precision float=w1017:dbl[])
                n490 = Index Array(array=w1017, index #1=0 ("index"), index #2=1 ("index")) -> (element #1=w1016:dbl, element #2=w1015:dbl)
                n491 = Divide(x=w1016, y=w1014) -> (x/y=w1013:dbl)
                n492 = Divide(x=w1015, y=w1014) -> (x/y=w1012:dbl)
                n493 = for {
                  tunnel: w1010 -> [w1024] mode=indexing
                  tunnel: w1013 -> [w1026]
                  tunnel: w1012 -> [w1025]
                  tunnel: w1011 -> [w1027]
                  n494 = property class="IntGraph (strict)"(reference=w1024, "Cursor.Visible"=w1027, "Cursor.Cursor X"=w1026, "Cursor.Cursor Y"=w1025) -> ()  [unwired: 1 in, 2 out]
                }
              }
              frame "Auto Scale" {
                n495 = Select(t=u8 2 ("Z Scale.Scale Fit"), s=w1031, f=u8 0) -> (s? t:f=w1028:u8)
                n496 = for {
                  tunnel: w1032 -> [w1034] mode=indexing
                  tunnel: w1028 -> [w1033]
                  n497 = property class="IntGraph (strict)"(reference=w1034, "ZScale.ScaleFit"=w1033) -> ()  [unwired: 1 in, 2 out]
                }
              }
              frame "Pan Tool", "Reset Zoom", "Zoom In", "Zoom Out" {
                n498 = case shown="\"Reset Zoom\"" w1042 {
                  tunnel: [0 ("Palette:Active Tool") 6 ("Palette:Active Tool") 7 ("Palette:Active Tool") 1 ("Palette:Active Tool") 0 ("Palette:Active Tool")] -> w1036
                  tunnel: w1035 -> [_ _ _ _ w1054]
                  frame Default {
                  }
                  frame "Zoom In" {
                  }
                  frame "Zoom Out" {
                  }
                  frame "Pan Tool" {
                  }
                  frame "Reset Zoom" {
                    n499 = property on="Reset Zoom" class="Bool (strict)"("Value"=FALSE) -> ()  [unwired: 2 in, 2 out]
                    n500 = for {
                      tunnel: w1054 -> [w1059] mode=indexing
                      tunnel: 5 ("Palette:Active Tool") -> [w1058]
                      n501 = property class="IntGraph (strict)"(reference=w1059, "ActPaletteTool"=w1058) -> ()  [unwired: 1 in, 2 out]
                    }
                  }
                }
                n502 = control-ref of="Zoom In"() -> (w1038:refnum<vi>)
                n503 = control-ref of="Zoom Out"() -> (w1040:refnum<vi>)
                n504 = control-ref of="Pan Tool"() -> (w1039:refnum<vi>)
                n505 = Build Array(w1038, w1040, w1039) -> (w1041:refnum<vi>[])
                n506 = for {
                  tunnel: w1041 -> [w1047] mode=indexing
                  tunnel: w1037 -> [w1045]
                  n507 = property class="Bool (strict)"(reference=w1047) -> (reference out=w1046:refnum<vi>, "Label.Text"=w1044:string)  [unwired: 1 in, 1 out]
                  n508 = Equal?(x=w1044, y=w1045) -> (x = y?=w1043:bool)
                  n509 = property class="Bool (strict)"(reference=w1046, "Value"=w1043) -> ()  [unwired: 1 in, 2 out]
                }
                n510 = for {
                  tunnel: w1035 -> [w1049] mode=indexing
                  tunnel: w1036 -> [w1048]
                  n511 = property class="IntGraph (strict)"(reference=w1049, "ActPaletteTool"=w1048) -> ()  [unwired: 1 in, 2 out]
                }
              }
              frame "Load File" {
                w1069 = u16 1 items=["Get Image", "Load and Read File"] ("Action")
                n512 = control-ref of="This VI"() -> (w1071:refnum<vi>)
                n513 = property on="Load File" class="Bool (strict)"("Value"=FALSE) -> ()  [unwired: 2 in, 2 out]
                n514 = call "GetDisplayClick.vi"("Display REFs In"=w1072, "Calling VI REF"=w1071) -> ("Display Index"=w1060:i32)  [unwired: 13 in]
                n515 = call "OpenDBL.vi"("Action"=w1069) -> ("Image"=w1068:sgl[], "Dimensions (Z, Y, X, t)"=w1067:i32[])  [unwired: 11 in, 2 out]
                n516 = Index Array(array=w1067, index #1=1 ("index"), index #2=2 ("index")) -> (element #1=w1064:i32, element #2=w1063:i32)
                n517 = Reverse 1D Array(array=w1068) -> (reversed array=w1062:sgl[])
                n518 = Reshape Array(w1062, w1064, w1063) -> (w1061:sgl[][])
                n519 = Index Array(array=w1072, index=w1060) -> (element=w1070:refnum<vi>)
                n520 = property class="IntGraph (strict)"(reference=w1070, "Value"=w1061) -> ()  [unwired: 1 in, 2 out]
              }
              frame "Fit Tool" {
                n521 = control-ref of="This VI"() -> (w1081:refnum<vi>)
                n522 = call "Image Aquisition Param Ctrl_AE.vi"("Action"=enum16{"READ", "WRITE"}."READ") -> ("Image Acquisition Parameters Out"=w1076:T17)  [unwired: 10 in]
                n523 = call "GetDisplayClick.vi"("Display REFs In"=w1079, "Calling VI REF"=w1081) -> ("Display Index"=w1080:i32)  [unwired: 13 in]
                n524 = Index Array(array=w1079, index=w1080) -> (element=w1078:refnum<vi>)
                n525 = property class="IntGraph (strict)"(reference=w1078) -> ("Value"=w1077:sgl[][])  [unwired: 1 in, 2 out]
                n526 = vi-ref "QuickProfile_V3.vi"() -> (w1084:refnum<vi>)
                n527 = property class="VI Interface Type 0"(reference=w1084) -> ("Path"=w1087:path)  [unwired: 1 in, 2 out]
                n528 = Unbundle By Name(w1076) -> ("Pixel Size (nm)"=w1083:dbl[])
                n529 = Index Array(array=w1083, index=0) -> (element=w1090:dbl)
                n530 = Open VI Reference(type specifier VI Refnum (for type only)=w1084, vi path=w1087, options=128) -> (vi reference=w1085:refnum<vi>)  [unwired: 3 in, 1 out]
                n531 = call-by-ref "Start Asynchronous Call"(reference=w1085, "Image IN"=w1077, "Pixel Size (nm)"=w1090) -> (reference out=w1088:refnum<vi>, error out=w1075:errorcluster)  [unwired: 15 in]
                n532 = Close Reference(reference=w1088) -> ()  [unwired: 1 in, 1 out]
                n533 = property on="Fit Tool" class="Bool (strict)"(error in=w1075, "Value"=FALSE) -> ()  [unwired: 1 in, 2 out]
              }
              frame "Smooth Tool" {
                n534 = vi-ref "SmoothTool.vi"() -> (w1095:refnum<vi>)
                n535 = property on="Smooth Tool" class="Bool (strict)"("Value"=FALSE) -> ()  [unwired: 2 in, 2 out]
                n536 = property class="VI Interface Type 1"(reference=w1095) -> ("Path"=w1097:path)  [unwired: 1 in, 2 out]
                n537 = control-ref of="This VI"() -> (w1093:refnum<vi>)
                n538 = Open VI Reference(type specifier VI Refnum (for type only)=w1095, vi path=w1097, options=128) -> (vi reference=w1096:refnum<vi>)  [unwired: 3 in, 1 out]
                n539 = call-by-ref "Start Asynchronous Call"(reference=w1096, "Calling VI REF"=w1093, "Display REFs In"=w1092) -> (reference out=w1094:refnum<vi>)  [unwired: 11 in, 1 out]
                n540 = Close Reference(reference=w1094) -> ()  [unwired: 1 in, 1 out]
              }
              frame "Merge Tool" {
                n541 = vi-ref "MergeTool - Cambridge.vi"() -> (w1103:refnum<vi>)
                n542 = property class="VI Interface Type 2"(reference=w1103) -> ("Path"=w1105:path)  [unwired: 1 in, 2 out]
                n543 = property on="Merge Tool" class="Bool (strict)"("Value"=FALSE) -> ()  [unwired: 2 in, 2 out]
                n544 = control-ref of="This VI"() -> (w1101:refnum<vi>)
                n545 = Open VI Reference(type specifier VI Refnum (for type only)=w1103, vi path=w1105, options=128) -> (vi reference=w1104:refnum<vi>)  [unwired: 3 in, 1 out]
                n546 = call-by-ref "Start Asynchronous Call"(reference=w1104, "VI Reference"=w1101, "Display References"=w1100) -> (reference out=w1102:refnum<vi>)  [unwired: 11 in, 1 out]
                n547 = Close Reference(reference=w1102) -> ()  [unwired: 1 in, 1 out]
              }
            }
          }
        }
      }
      event "Channel 1", "Channel 2", "Channel 3", "Channel 4", "Channel 5", "Channel 6": Mouse Down; "Channel 1", "Channel 2", "Channel 3", "Channel 4", "Channel 5", "Channel 6": Mouse Up {
        n548 = event-data() -> ("Type"=w1112:T28, "CtlRef"=w1109:refnum<vi>)  [unwired: 1 in, 5 out]
        n549 = Equal?(x=w1112, y=lveventtype."Mouse Down" ("Type")) -> (x = y?=w1110:bool)
        n550 = call "Graph Ref AE.vi"("Action"=enum16{"READ", "WRITE"}."READ") -> ("Graph Ref Out"=w1107:refnum<vi>[])  [unwired: 10 in]
        n551 = case shown="True" w1110 {
          tunnel: w1109 -> [w1115 w1133]
          tunnel: w1107 -> [w1114 w1132]
          frame False {
            n552 = property class="IntGraph (strict)"(reference=w1115) -> (reference out=w1119:refnum<vi>, "ActPaletteTool"=w1116:i32)  [unwired: 1 in, 1 out]
            n553 = Not Equal?(x=w1116, y=0) -> (x != y?=w1118:bool)
            n554 = case shown="False" w1118 {
              tunnel: w1119 -> [w1122 w1128]
              tunnel: w1114 -> [w1121 w1125]
              frame False {
                n555 = property class="IntGraph (strict)"(reference=w1122) -> ("Cursor.Cursor Position"=w1120:T42)  [unwired: 1 in, 2 out]
                n556 = for {
                  tunnel: w1121 -> [w1123] mode=indexing
                  tunnel: w1120 -> [w1124]
                  n557 = property class="IntGraph (strict)"(reference=w1123, "Cursor.Cursor Position"=w1124) -> ()  [unwired: 1 in, 2 out]
                }
              }
              frame True {
                n558 = property class="IntGraph (strict)"(reference=w1128) -> ("XScale.Range"=w1127:T43, "YScale.Range"=w1126:T43)  [unwired: 1 in, 2 out]
                n559 = for {
                  tunnel: w1127 -> [w1131]
                  tunnel: w1126 -> [w1130]
                  tunnel: w1125 -> [w1129] mode=indexing
                  n560 = property class="IntGraph (strict)"(reference=w1129, "XScale.Range"=w1131, "YScale.Range"=w1130) -> ()  [unwired: 1 in, 2 out]
                }
              }
            }
          }
          frame True {
            n561 = for {
              tunnel: w1132 -> [w1138] mode=indexing
              tunnel: w1133 -> [w1139]
              n562 = Equal?(x=w1138, y=w1139) -> (x = y?=w1137:bool)
              n563 = Select(t=T29 {"Left"=2431, "Top"=-324} ("Z Scale.Position"), s=w1137, f=T29 {"Left"=0, "Top"=0}) -> (s? t:f=w1134:T29)
              n564 = property class="IntGraph (strict)"(reference=w1138, "ZScale.Visible"=w1137, "ZScale.Position"=w1134) -> ()  [unwired: 1 in, 2 out]
            }
          }
        }
      }
      event "Exit": Value Change {
        n565 = event-data() -> ("CtlRef"=w1164:refnum<vi>, "NewVal"=w1166:bool)  [unwired: 1 in, 1 out]
        n566 = Release Notifier(notifier=w1159, force destroy? (F)=TRUE) -> ()  [unwired: 1 in, 3 out]
        n567 = property class="Bool"(reference=w1164) -> ("Label.Text"=w1163:string)  [unwired: 1 in, 2 out]
        n568 = call "SLM AE.vi"("Action"=enum16{"READ", "WRITE"}."READ") -> ("SLM Ref Out"=w1157:refnum<vi>)  [unwired: 10 in]
        n569 = call "DM_Ref_AE.vi"("Action"=enum16{"READ", "WRITE"}."READ") -> ("DM Ref Out"=w1155:refnum<vi>)  [unwired: 10 in]
        n570 = call "GateDelay AE.vi"("Action"=enum16{"READ", "WRITE"}."READ") -> ("Gate Delay Ref Out"=w1156:refnum<vi>)  [unwired: 10 in]
        n571 = Enqueue Element(queue=w1165, element=w1163) -> ()  [unwired: 2 in, 3 out]
        n572 = Build Array(w1157, w1155, w1156) -> (w1154:refnum<vi>[])
        n573 = call "Stage_position_ae.vi"("StageID"="N664", "Enum"=enum16{"WRITE", "READ", "HOME", "SAVE HOME"}."HOME") -> ("Position Out"=w1146:dbl[])  [unwired: 8 in, 1 out]
        n574 = call "Stage_position_ae.vi"("StageID"="P541", "Enum"=enum16{"WRITE", "READ", "HOME", "SAVE HOME"}."HOME") -> ("Position Out"=w1150:dbl[])  [unwired: 8 in, 1 out]
        n575 = for {
          tunnel: w1154 -> [w1171] mode=indexing
          n576 = Not A Number/Path/Refnum?(number/path/refnum=w1171) -> (NaN/Path/Refnum?=w1170:bool)
          n577 = case shown="False" w1170 {
            tunnel: w1171 -> [w1172 _]
            frame False {
              n578 = To Variant(anything=TRUE) -> (Variant=w1173:variant)
              n579 = invoke class="VI" method="Ctrl Val.Set"(reference=w1172, "Control Name"="Exit", "Value"=w1173) -> (reference out=w1176:refnum<vi>)  [unwired: 2 in, 4 out]
              n580 = Close Reference(reference=w1176) -> ()  [unwired: 1 in, 1 out]
            }
            frame True {
            }
          }
        }
        n581 = Index Array(array=w1146, index=0) -> (element=w1143:dbl)
        n582 = property on="Stages" class="Clust (strict)"() -> ("Controls[]"=w1153:refnum<vi>[])  [unwired: 2 in, 2 out]
        n583 = Index Array(array=w1150, index=0) -> (element=w1144:dbl)
        n584 = Build Array(w1144, w1143) -> (w1142:dbl[])
        n585 = for {
          tunnel: w1153 -> [w1169] mode=indexing
          n586 = property class="Ctl"(reference=w1169) -> ("Label.Text"=w1168:string)  [unwired: 1 in, 2 out]
          n587 = call "All_Stages_Aloha.vi"("Aloha"=FALSE, "Stage ID"=w1168) -> ()  [unwired: 9 in, 1 out]
        }
        n588 = call-poly <vilib>:"Write To Spreadsheet File.vi"("format (%.3f)"="%.4f", "1D data"=w1142, "file path (dialog if empty)"=path "C:/Users/ED STED/Documents/Test Control Software/Host VIs/Stages/Stage Positions/home position.csv") -> ()  [unwired: 5 in, 1 out]
      }
    }
  }
  n589 = call "Manual Controls Action Engine.vi"("Action"=enum16{"Read", "Write"}."Write", "Manual Controls In"=w27) -> ("Manual Controls Out"=w29:T19)  [unwired: 13 in]
  n590 = call "FPGA-7842R-Control V2.vi"("Action"=FPGA-7842R-Reference."Initialize", "Manual Controls"=w29, "Initialize"=FALSE) -> ("Initalized"=w11:bool)  [unwired: 11 in, 1 out]
  n591 = while {
    shift-right: [w1189] -> _
    shift-left: "Idle" -> [w1190]
    tunnel: w18 -> [w1186]
    shift-right: [w1184] -> _
    shift-left: w11 -> [w1185]
    tunnel: w1 -> [w1177]
    stop <- w1188 stop-if-true
    n592 = call "Image Aquisition Param Ctrl_AE.vi"("Action"=enum16{"READ", "WRITE"}."READ") -> ("Image Acquisition Parameters Out"=w1183:T17)  [unwired: 10 in]
    n593 = call "Detectors Crl_AE.vi"("Action"=enum16{"READ", "WRITE"}."READ") -> ("Detectors Parameters Out"=w1181:T15)  [unwired: 10 in]
    n594 = call "Manual Controls Action Engine.vi"("Action"=enum16{"Read", "Write"}."Read") -> ("Manual Controls Out"=w1178:T19)  [unwired: 14 in]
    n595 = case shown="\"Stop Acquisition\"" w1190 {
      selector: w1190 -> [_ _ _ w1223 _ _ _ _ _ _]
      tunnel: ["Exit" w1199 "Idle" ("name (unnamed)") "Arange Displays" ("name (unnamed)") "Start FPGA Acquisition" ("name (unnamed)") "Display" ("name (unnamed)") "Close Images" ("name (unnamed)") "Idle" "Stop Waveforms" ("name (unnamed)") "Start Waveforms" ("name (unnamed)")] -> w1189
      tunnel: [TRUE w1201 w1208 w1231 w1249 w1273 w1314 w1347 w1356 w1394] -> w1188
      tunnel: FALSE -> [_ w1201 w1208 w1231 w1249 w1273 w1314 w1347 w1356 w1394]
      tunnel: w1186 -> [_ w1200 _ _ _ _ _ _ _ _]
      tunnel: w1185 -> [w1195 w1198 w1209 w1229 w1246 w1271 w1312 w1345 w1348 w1395]
      tunnel: [w1194 w1198 w1209 w1229 w1246 w1267 w1312 w1344 w1348 w1395] -> w1184
      tunnel: w1183 -> [_ _ _ w1222 _ w1266 _ _ _ w1392]
      tunnel: w1181 -> [_ _ _ w1221 _ _ _ _ _ w1390]
      tunnel: w1178 -> [_ _ _ w1212 _ _ _ _ _ _]
      tunnel: w1177 -> [_ _ _ _ w1239 _ _ _ _ _]
      frame "Exit" {
        n596 = call "Graph Ref AE.vi"("Action"=enum16{"READ", "WRITE"}."READ") -> ("Graph Ref Out"=w1192:refnum<vi>[])  [unwired: 10 in]
        n597 = call "FPGA-7842R-Control V2.vi"("Action"=FPGA-7842R-Reference."Close FPGA", "Initialize"=w1195) -> ("Initalized"=w1194:bool)  [unwired: 12 in, 1 out]
        n598 = Close Reference(reference=w1192) -> ()  [unwired: 1 in, 1 out]
      }
      frame "Idle", Default {
        n599 = Dequeue Element(queue=w1200, timeout in ms (-1)=-1) -> (element=w1199:string)  [unwired: 1 in, 3 out]
      }
      frame "Close Images" {
        w1204 = u16 0 items=["Read", "Write"] ("Mode")
        w1205 = u16 0 items=["Write", "Read"] ("Mode")
        n600 = call "File Action V1.vi"("Mode"=w1204) -> ("Files Open"=w1203:bool)  [unwired: 12 in, 2 out]
        n601 = call "Image_Actions_V1.vi"("Mode"=w1205, "Action"="Trash Images") -> ()  [unwired: 12 in, 2 out]
        n602 = case shown="True" w1203 {
          frame False {
          }
          frame True {
            w1211 = u16 1 items=["Read", "Write"] ("Mode")
            n603 = call "File Action V1.vi"("Action"="Close Files", "Mode"=w1211) -> ()  [unwired: 11 in, 3 out]
          }
        }
      }
      frame "Capture", "Live" {
        w1227 = u16 0 items=["Write", "Read"] ("Mode")
        n604 = Cluster To Array(cluster=w1221) -> (array=w1219:bool[])
        n605 = Index Array(array=w1219, index=4) -> (element=w1216:bool)
        n606 = Boolean To (0,1)(Boolean=w1219) -> (0, 1=w1220:i16[])
        n607 = Add Array Elements(numeric array=w1220) -> (sum=w1217:i16)
        n608 = To Long Integer(number=w1217) -> (32bit integer=w1214:i32)
        n609 = Unbundle By Name(w1222) -> ("Image Format"=w1224:u16)
        n610 = Select(t=1, s=w1216, f=w1214) -> (s? t:f=w1213:i32)
        n611 = case shown="\"Capture\"" w1223 {
          tunnel: w1222 -> [_ w1234]
          tunnel: w1213 -> [_ w1233]
          tunnel: w1212 -> [_ w1232]
          frame Default {
          }
          frame "Capture" {
            w1237 = u16 1 items=["Read", "Write"] ("Mode")
            n612 = call "File Action V1.vi"("Action"="Open Files", "Mode"=w1237, "Image Acquisition Parameters"=w1234, "Manual Controls In"=w1232, "File Path IN"="Save File Path", "Number of Channels"=w1233) -> ("File Path OUT"=w1235:path)  [unwired: 7 in, 2 out]
            n613 = local write "Save File Path"(w1235) -> ()
          }
        }
        n614 = To Long Integer(number=w1224) -> (32bit integer=w1226:i32)
        n615 = Bundle(w1226, w1226) -> (w1225:cluster{i32, i32})  [unwired: 1 in]
        n616 = call "Image_Actions_V1.vi"("Image Size (Pixels)"=w1225, "Mode"=w1227, "Number of Channels"=w1213, "Action"="Create Images") -> ()  [unwired: 10 in, 2 out]
      }
      frame "Arange Displays" {
        w1244 = u16 1 items=["Write", "Read"] ("Mode")
        w1247 = u16 1 items=["Read", "Write"] ("Action")
        n617 = call "Image_Actions_V1.vi"("Mode"=w1244) -> ("Image REFs OUT"=w1245:T44[])  [unwired: 13 in, 1 out]
        n618 = call "Graph Ref AE.vi"("Action"=enum16{"READ", "WRITE"}."READ", "Graph Ref In"=w1239) -> ("Graph Ref Out"=w1241:refnum<vi>[])  [unwired: 9 in]
        n619 = Array Size(array=w1245) -> (size(s)=w1243:i32)
        n620 = call "Arange_Displays_V2.vi"("Display References"=w1241, "Action"=w1247, "Number of Channels"=w1243, "Aspect Ratio (h/w)"=1.0) -> ("Number of Channels OUT"=w1242:i32)  [unwired: 11 in]
        n621 = for {
          N: w1242 -> [_]
          tunnel: w1241 -> [w1251] mode=indexing
          tunnel: [w1254] -> _ mode=indexing
          i -> [w1252]
          n622 = property class="IntGraph (strict)"(reference=w1251) -> ("Label.Text"=w1256:string)  [unwired: 1 in, 2 out]
          n623 = Equal To 0?(x=w1252) -> (x = 0?=w1253:bool)
          n624 = case shown="True" w1253 {
            tunnel: w1251 -> [_ w1257]
            frame False {
            }
            frame True {
              n625 = property class="IntGraph (strict)"(reference=w1257, "ZScale.Visible"=TRUE ("Z Scale.Visible"), "ZScale.Position"=T29 {"Left"=2431, "Top"=-324} ("Z Scale.Position")) -> ()  [unwired: 1 in, 2 out]
            }
          }
          n626 = To Unsigned Word Integer(number=w1252) -> (unsigned 16bit integer=w1255:u16)
          n627 = Bundle("Label.Text"=w1256, w1255) -> (w1254:cluster{"Label.Text":string, u16})  [unwired: 1 in]
        }
        "Graph Ref Out" <- w1239
      }
      frame "Start Waveforms" {
        n628 = Unbundle By Name("Laser Controls 2") -> ("Laser On Time (Ticks)"=w1261:i8, "Laser Delay (Ticks)"=w1260:i8)
        n629 = call "Initialize Waveforms V4.vi"("Image Acquisition Parameters"=w1266) -> ("Waveform Data to FPGA"=w1272:T45)  [unwired: 14 in]
        n630 = Unbundle By Name(w1266) -> ("Scan Type"=w1265:enum16{"Sample Scanning", "Beam Scanning"})
        n631 = call "FPGA-7842R-Control V2.vi"("Waveform Data"=w1272, "Action"=FPGA-7842R-Reference."Start Waveforms", "Laser On Time (Ticks)"=w1261, "Image Acquisition Parameters"=w1266, "Initialize"=w1271, "Laser Delay (Ticks)"=w1260) -> ("Initalized"=w1268:bool)  [unwired: 8 in, 1 out]
        n632 = Equal?(x=w1265, y=enum16{"Sample Scanning", "Beam Scanning"}."Sample Scanning" ("Scan Type")) -> (x = y?=w1263:bool)
        n633 = case shown="True" w1263 {
          tunnel: w1268 -> [w1274 w1279]
          tunnel: [w1274 w1278] -> w1267
          frame False {
          }
          frame True {
            n634 = call "Scan Parameters Action Engine.vi"("Action"=enum16{"Read", "Write"}."Read") -> ("Scan Parameters OUT"=w1276:T18)  [unwired: 14 in]
            n635 = Unbundle By Name(w1276) -> ("Unused_Axis_I16"=w1275:i16)
            n636 = call "FPGA-7842R-Control V2.vi"("Action"=FPGA-7842R-Reference."Unused Axis I16", "Initialize"=w1279, "Unused Axis Offset (I16)"=w1275) -> ("Initalized"=w1278:bool)  [unwired: 11 in, 1 out]
          }
        }
      }
      frame "Display" {
        w1307 = u16 1 items=["Write", "Read"] ("Mode")
        n637 = call "Image_Actions_V1.vi"("Mode"=w1307) -> ("Image REFs OUT"=w1309:T44[])  [unwired: 13 in, 1 out]
        n638 = Array Size(array=w1309) -> (size(s)=w1305:i32)
        n639 = Decrement(x=w1305) -> (x-1=w1304:i32)
        n640 = for {
          N: 6 -> [_]
          tunnel: w1304 -> [w1342]
          tunnel: [w1340] -> w1308 mode=indexing
          i -> [w1341]
          n641 = Greater Or Equal?(x=w1342, y=w1341) -> (x >= y?=w1340:bool)
        }
        n642 = Obtain Notifier(name (unnamed)="Running", notification data type=FALSE) -> (notifier out=w1281:refnum<notifier>)  [unwired: 2 in, 2 out]
        n643 = Index Array(array=w1308, index #1=1 ("index"), index #2=2 ("index"), index #3=3 ("index"), index #4=4 ("index"), index #5=5 ("index")) -> (element #1=w1293:bool, element #2=w1292:bool, element #3=w1291:bool, element #4=w1290:bool, element #5=w1289:bool)
        n644 = Index Array(array=w1309, index #1=0 ("index"), index #2=1 ("index"), index #3=2 ("index"), index #4=3 ("index"), index #5=4 ("index"), index #6=5 ("index")) -> (element #1=w1288:T44, element #2=w1287:T44, element #3=w1286:T44, element #4=w1285:T44, element #5=w1284:T44, element #6=w1283:T44)
        n645 = while {
          tunnel: w1293 -> [w1329]
          tunnel: w1292 -> [w1328]
          tunnel: w1291 -> [w1324]
          tunnel: w1290 -> [w1321]
          tunnel: w1289 -> [w1320]
          tunnel: w1288 -> [w1327]
          tunnel: w1287 -> [w1326]
          tunnel: w1286 -> [w1325]
          tunnel: w1285 -> [w1323]
          tunnel: w1284 -> [w1319]
          tunnel: w1283 -> [w1322]
          tunnel: w1281 -> [w1316]
          stop <- w1317 stop-if-true
          n646 = Get Notifier Status(notifier=w1316) -> (current notification=w1317:bool)  [unwired: 1 in, 4 out]
          n647 = case shown="False" w1329 {
            tunnel: w1326 -> [_ w1339]
            frame False {
            }
            frame True {
              n648 = call "IMAQ ImageToArray"("Image"=w1339) -> ("Image Pixels (Float)"=→"Channel 2":sgl[][])  [unwired: 3 in, 4 out]
            }
          }
          n649 = case shown="False" w1328 {
            tunnel: w1325 -> [_ w1337]
            frame False {
            }
            frame True {
              n650 = call "IMAQ ImageToArray"("Image"=w1337) -> ("Image Pixels (Float)"=→"Channel 3":sgl[][])  [unwired: 3 in, 4 out]
            }
          }
          n651 = call "IMAQ ImageToArray"("Image"=w1327) -> ("Image Pixels (Float)"=→"Channel 1":sgl[][])  [unwired: 3 in, 4 out]
          n652 = case shown="False" w1324 {
            tunnel: w1323 -> [_ w1335]
            frame False {
            }
            frame True {
              n653 = call "IMAQ ImageToArray"("Image"=w1335) -> ("Image Pixels (Float)"=→"Channel 4":sgl[][])  [unwired: 3 in, 4 out]
            }
          }
          n654 = case shown="False" w1321 {
            tunnel: w1319 -> [_ w1333]
            frame False {
            }
            frame True {
              n655 = call "IMAQ ImageToArray"("Image"=w1333) -> ("Image Pixels (Float)"=→"Channel 5":sgl[][])  [unwired: 3 in, 4 out]
            }
          }
          n656 = case shown="False" w1320 {
            tunnel: w1322 -> [_ w1331]
            frame False {
            }
            frame True {
              n657 = call "IMAQ ImageToArray"("Image"=w1331) -> ("Image Pixels (Float)"=→"Channel 6":sgl[][])  [unwired: 3 in, 4 out]
            }
          }
          n658 = Wait (ms)(milliseconds to wait=u32 100) -> ()  [unwired: 1 out]
        }
      }
      frame "Stop Waveforms" {
        n659 = call "FPGA-7842R-Control V2.vi"("Action"=FPGA-7842R-Reference."Stop Waveforms", "Initialize"=w1345) -> ("Initalized"=w1344:bool)  [unwired: 12 in, 1 out]
      }
      frame "Stop Acquisition" {
        n660 = call "FPGA-7842R-Control V2.vi"("Action"=FPGA-7842R-Reference."Laser Control", "Laser Controls"=T16 {"STED Power (V)"=0.0, "STED"=FALSE, "650 nm"=FALSE, "590 nm"=FALSE, "485 nm"=FALSE, "Manual Control"=FALSE} ("Laser Controls 2"), "Initialize"=TRUE) -> ()  [unwired: 11 in, 2 out]
        n661 = call "AO AE.vi"("Action"=enum16{"READ", "WRITE"}."READ") -> ("Z Comp. Output"=w1350:T1)  [unwired: 8 in, 2 out]
        n662 = Unbundle By Name(w1350) -> ("Enable"=w1349:bool)
        n663 = case shown="True" w1349 {
          frame False {
          }
          frame True {
            n664 = call "Image Aquisition Param Ctrl_AE.vi"("Action"=enum16{"READ", "WRITE"}."READ") -> ("Image Acquisition Parameters Out"=w1360:T17)  [unwired: 10 in]
            n665 = Unbundle By Name(w1360) -> ("Scan Mode"=w1359:enum16{"XY", "XZ", "YZ", "XYZ"})
            n666 = Equal?(x=w1359, y=enum16{"XY", "XZ", "YZ", "XYZ"}."XYZ") -> (x = y?=w1357:bool)
            n667 = case shown="True" w1357 {
              frame False {
              }
              frame True {
                w1364 = 1 ("disabled index (col)")
                w1366 = 0 ("disabled index (col)")
                n668 = call "AO AE.vi"("Action"=enum16{"READ", "WRITE"}."READ") -> ("Mirror Modes Out"=w1368:T36, "DM Value Output"=w1371:dbl[][], "Z Comp. Output"=w1382:T1)  [unwired: 8 in]
                n669 = call "Mirror_Mode_DUAL_AE.vi"("Action"=Standard_Action."Write", "Mirror Modes In"=w1368) -> ()  [unwired: 13 in, 1 out]
                n670 = call "Deform_Mirror_DUAL_AE_V2.vi"("Action"=Standard_Action."Read") -> ("Refnum Out"=w1376:refnum<k7>, "Multi Map Data Out"=w1374:i32[])  [unwired: 10 in, 3 out]
                n671 = Index Array(array=w1371, index (col)=w1366) -> (element=w1367:dbl[])  [unwired: 1 in]
                n672 = Unbundle By Name(w1382) -> ("Origin (um)"=w1385:dbl)
                n673 = call "Voltage vs Signal_Data Engine_V1.vi"("Control Signal In (-1~1)"=w1367, "DM #"=w1366) -> ("Voltage Out (0~Max. Vol.)"=w1365:dbl[])  [unwired: 1 in, 1 out]
                n674 = control-ref of="Abort AllStage"() -> (w1378:refnum<vi>)
                n675 = call "WriteDM_V2.vi"("reference in"=w1376, "nDevId"=0, "MultiDM  Mapping"=w1374, "Voltage Array in"=w1365) -> ("reference out"=w1375:refnum<k7>)  [unwired: 2 in, 1 out]
                n676 = Build Array(w1385) -> (w1384:dbl[])
                n677 = Bundle By Name(cluster=w1382, "Enable"=FALSE) -> (w1380:T1)
                n678 = Index Array(array=w1371, index (col)=w1364) -> (element=w1363:dbl[])  [unwired: 1 in]
                n679 = call "AE_AllStages_Action V2.vi"("Velocity"=10000.0, "Abort"=w1378, "Positions"=w1384, "Axis"=bool[] [TRUE], "Stage ID"="P841", "Action"=StageStates."MOVE") -> ()  [unwired: 3 in, 3 out]
                n680 = call "Voltage vs Signal_Data Engine_V1.vi"("Control Signal In (-1~1)"=w1363, "DM #"=w1364) -> ("Voltage Out (0~Max. Vol.)"=w1362:dbl[])  [unwired: 1 in, 1 out]
                n681 = call "WriteDM_V2.vi"("reference in"=w1375, "nDevId"=1, "MultiDM  Mapping"=w1374, "Voltage Array in"=w1362) -> ()  [unwired: 2 in, 2 out]
                n682 = call "AO AE.vi"("Mirror Modes In"=w1368, "DM Value Input"=w1371, "Z Comp. Input"=w1380, "Action"=enum16{"READ", "WRITE"}."WRITE") -> ()  [unwired: 5 in, 3 out]
                n683 = call "Pixel Value (-1 to 1) DUAL AE.vi"("Action"=Standard_Action."Write", "Pixel Value (-1 to 1)"=w1371) -> ()  [unwired: 13 in, 1 out]
              }
            }
          }
        }
      }
      frame "Start FPGA Acquisition" {
        n684 = Unbundle By Name(w1392) -> ("Scan Mode"=w1391:enum16{"XY", "XZ", "YZ", "XYZ"})
        n685 = case shown="\"XZ\", Default" w1391 {
          tunnel: w1392 -> [_ w1403]
          tunnel: w1390 -> [_ w1402]
          frame "YZ" {
            n686 = vi-ref "FPGA Sample Scanning V1.vi"() -> (w1398:refnum<vi>)
            n687 = property class="VI Interface Type 3"(reference=w1398) -> ("Path"=w1396:path)  [unwired: 1 in, 2 out]
            n688 = Open VI Reference(type specifier VI Refnum (for type only)=w1398, vi path=w1396, options=128) -> (vi reference=w1399:refnum<vi>)  [unwired: 3 in, 1 out]
            n689 = call-by-ref "Start Asynchronous Call"(reference=w1399) -> (reference out=w1400:refnum<vi>)  [unwired: 4 in, 1 out]
            n690 = Close Reference(reference=w1400) -> ()  [unwired: 1 in, 1 out]
          }
          frame "XZ", Default {
            n691 = vi-ref "FPGA Beam Scanning V2.vi"() -> (w1405:refnum<vi>)
            n692 = property class="VI Interface Type 4"(reference=w1405) -> ("Path"=w1406:path)  [unwired: 1 in, 2 out]
            n693 = Open VI Reference(type specifier VI Refnum (for type only)=w1405, vi path=w1406, options=128) -> (vi reference=w1404:refnum<vi>)  [unwired: 3 in, 1 out]
            n694 = call-by-ref "Start Asynchronous Call"(reference=w1404, "Detectors"=w1402, "Image Acquisition Parameters"=w1403) -> (reference out=w1401:refnum<vi>)  [unwired: 3 in, 1 out]
            n695 = Close Reference(reference=w1401) -> ()  [unwired: 1 in, 1 out]
          }
        }
      }
    }
  }
